vi "Tetra_TX-ATTEN_Payload.vi"(8 "error in":errorcluster, 10 "Input Constants":string[](array[string])=["18.75;1", "5;1", "COM4", "1", "1", "25", "0;0", "0;0", "1;20", "0", "0", "0", "", "10", "Z:\\State Files\\TEST2.csa", "", "3000", "4", "-10", "0.1", "", "", "C:\\RageATE\\Automated Tests\\Tetra WAM\\DVT\\Cal Files\\OUTPUT_CAL_080321-1118.csv"], 11 "Parameters":string[](array[string])=["skip", "18.75", "1", "5", "-1", "0", "5", "32.900000"]) -> (0 "error out":errorcluster, 2 "Payload Results":string[](array[string])=["-1.000", "-1.000", "32900.031", "-94.423", "-86.423", "-1.000", "16.450", "-1.000", "-1.000", "-1.000", "-1.000", "-1.000", "3.000", "-1.000", "-1.000", "15.000", "8.000", "8.000", "8.000", "-1.000", "-1.000", "-1.000", "-1.000", "-1.000", "-1.000", "-1.000", "-1.000", "-1.000", "-1.000", "-1.000", "-1.000", "-1.000", "-1.000", "-1.000", "-1.000", "-1.000", "-1.000", "-1.000", "-1.000", "-1.000", "-1.000", "-1.000", "-1.000", "-1.000", "0.504", "130.000", "-8.000", "32900.000", "-1.000", "-1.000", "P0027", "", "-1"])   [LabVIEW 2018]
uses:
  C:/RageATE-Tetra/Instruments/Ess Temp Plate/LabView Driver/Public/Watbus.dll
  Instruments/Ess Temp Plate/LabView Driver/Public/Watbus.dll
  8a334051-eedf-4406-ba3b-4766be56bf9e.vi
  458b4a15-084f-46bd-ad65-8d84519d0715.vi
  e7e3a4d5-9ed6-4285-8f90-f7af1205463a.vi
  778a857b-ea1c-4c41-85f0-8bde546241f8.vi
  765396e5-d7fa-4d1d-a6be-20604e030d46.vi
  35825170-2933-49a7-a6a3-6a45a8b9c174.vi
  498168d9-979f-4171-bbb2-b986919cd012.vi
  fd570da2-80e1-4258-b5ac-03cfe2f2c2d7.vi
  51f53847-2d88-46b1-9baf-ea88b261c08d.vi
  Initialize References/Station References Global.vi
  Initialize References/Sequence Globals.vi
  Tetra_Globals.vi
  Infrastructure/Test Parameter Globals_1.0.0.vi
  <vilib>/Utility/file.llb/Write Delimited Spreadsheet (DBL).vi
  <vilib>/Utility/file.llb/Read Delimited Spreadsheet (DBL).vi
  Instruments/Agilent N5232A PNA-L/Labview Driver/Keysight PNA Series/Keysight PNA Series.lvlib
  Instruments/PNA/lib functions/Agilent ENA Series.lvlib
panel:
  out "support_path":path
  out "RevC(t)":bool
  out "use-psa(t)":bool
  out "use-adar(t)":bool
  out "imon_pass?(t)":bool
  out "att_inl":dbl
  out "att_ref":dbl
  out "FiltRead":bool
  out "fault?(t)":bool
  in  "ess_error":errorcluster
  out "Freq Display":dbl=32.9 caption="Freq :  20"
  in  "Tab Control":T1(tab)
  out "MEAS_DCMON":bool
  out "CHIP_TEMP(t)":bool
  out "COMPORT":string="COM4"
  out "MODE":bool=TRUE
  out "Dist":dbl
  out "FILT_FCUT":dbl=25.0
  out "PLATE_TEMP(t)":bool
  out "MEAS_PS":bool
  out "MEAS_H2":bool=TRUE
  out "MEAS_Hx":bool=TRUE
  out "Hx_FREQ":dbl
  out "Hx_MULT":dbl
  out "H2_FREQ":dbl=40.0
  out "GANTRY(t)":bool=TRUE
  out "GET_DETECT":bool
  out "cmd;":string
  out "SOAK(m)":dbl
  out "Apply_FSL(t)":bool=TRUE
  out "MEAS_S11":bool
  out "S11_PORT":dbl
  out "comport":refnum<visa-resource-name>="COM4"
  out "AVG":i32=4
  out "ILabVIEW":refnum<k24>
  out "TEMP":dbl=25.0
  out "TX_PORT":i32=1
  out "V_SUPPLY":dbl=18.75
  out "EXT_ATT":dbl=5.0
  out "ADAR ATT":dbl
  out "TX_FILTER":i32=3
  out "REF_POW":dbl=5.0
  out "RF_FREQ":dbl=32.9
  out "TEMP(t)":bool
  out "V_SUPPLY(t)":bool
  out "TX_PORT(t)":bool
  out "REF_PWR(t)":bool
  out "TX_FILT(t)":bool
  out "ADAR_ATT(t)":bool
  out "EXT_ATT(t)":bool
  out "RF_FREQ(t)":bool=TRUE
  out "f_ref":dbl=16.45
  out "hx(t)":bool
  out "h2(t)":bool
  out "ps_meas(i)(w)":dbl[](array[numeric])=[-1.0, -1.0]
  out "rdv":dbl[](array[numeric])=[-1.0, -1.0, -1.0, -1.0, -1.0, -1.0, -1.0, -1.0, -1.0, -1.0]
  out "rdiv(i)":dbl[](array[numeric])=[-1.0, -1.0, -1.0, -1.0, -1.0, -1.0]
  out "rdiv(v)":dbl[](array[numeric])=[-1.0, -1.0, -1.0, -1.0, -1.0, -1.0]
  out "exa_mkr":dbl[](array[numeric])=[32900.0309, -94.423]
  out "h2_mkr":dbl[](array[numeric])=[-1.0, -1.0]
  out "Ampl_corr":dbl=-86.423
  out "s11":dbl=-1.0
  out "fsl_ampl_corr":dbl
  out "out_cal_ampl":dbl=-8.0
  out "out_cal freq":dbl=32900.0
  out "h2_dbc":dbl=-1.0
  out "hx_dbc":dbl
  out "hx_mkr":dbl[](array[numeric])
  out "fsl_corr_dB":dbl
  out "fsl(dB)":dbl
  out "att_dnl":dbl
  out "h2_lim":dbl
  out "out_cal":dbl[][](array[numeric])=[[0.0, 0.0], [20000.0, -6.076], [20100.0, -6.075], [20200.0, -6.219], [20300.0, -6.234], [20400.0, -6.315], [20500.0, -6.131], [20600.0, -6.004], [20700.0, -6.283], [20800.0, -6.485], [20900.0, -6.42], [21000.0, -6.941], [21100.0, -6.789], [21200.0, -6.508], [21300.0, -6.41], [21400.0, -6.872], [21500.0, -6.938], [21600.0, -7.017], [21700.0, -7.269], [21800.0, -6.683], [21900.0, -6.297], [22000.0, -6.38], [22100.0, -6.432], [22200.0, -6.851], [22300.0, -6.503], [22400.0, -6.961], [22500.0, -6.827], [22600.0, -6.62], [22700.0, -6.74], [22800.0, -6.547], [22900.0, -6.559], [23000.0, -6.434], [23100.0, -6.642], [23200.0, -6.654], [23300.0, -6.563], [23400.0, -6.6], [23500.0, -6.836], [23600.0, -6.685], [23700.0, -6.139], [23800.0, -6.472], [23900.0, -6.849], [24000.0, -6.765], [24100.0, -6.802], [24200.0, -6.636], [24300.0, -6.397], [24400.0, -6.33], [24500.0, -6.799], [24600.0, -6.985], [24700.0, -7.181], [24800.0, -7.304], [24900.0, -7.242], [25000.0, -7.104], [25100.0, -7.249], [25200.0, -7.246], [25300.0, -7.161], [25400.0, -7.073], [25500.0, -7.471], [25600.0, -7.347], [25700.0, -7.254], [25800.0, -7.048], [25900.0, -7.016], [26000.0, -7.055], [26100.0, -7.436], [26200.0, -7.416], [26300.0, -7.406], [26400.0, -7.616], [26500.0, -7.56], [26600.0, -7.304], [26700.0, -7.165], [26800.0, -7.047], [26900.0, -7.196], [27000.0, -8.144], [27100.0, -7.775], [27200.0, -7.683], [27300.0, -8.261], [27400.0, -7.702], [27500.0, -7.067], [27600.0, -7.418], [27700.0, -7.363], [27800.0, -7.557], [27900.0, -8.241], [28000.0, -7.789], [28100.0, -7.932], [28200.0, -7.422], [28300.0, -7.539], [28400.0, -7.363], [28500.0, -7.293], [28600.0, -7.623], [28700.0, -7.8], [28800.0, -7.603], [28900.0, -7.302], [29000.0, -7.428], [29100.0, -7.212], [29200.0, -7.395], [29300.0, -7.337], [29400.0, -7.17], [29500.0, -7.328], [29600.0, -7.393], [29700.0, -7.363], [29800.0, -7.396], [29900.0, -7.295], [30000.0, -7.448], [30100.0, -7.434], [30200.0, -7.524], [30300.0, -7.411], [30400.0, -7.422], [30500.0, -7.643], [30600.0, -7.707], [30700.0, -7.612], [30800.0, -7.742], [30900.0, -7.916], [31000.0, -7.904], [31100.0, -8.064], [31200.0, -8.185], [31300.0, -8.079], [31400.0, -8.102], [31500.0, -8.357], [31600.0, -7.974], [31700.0, -8.361], [31800.0, -8.902], [31900.0, -8.745], [32000.0, -8.522], [32100.0, -8.392], [32200.0, -8.221], [32300.0, -7.885], [32400.0, -8.215], [32500.0, -8.486], [32600.0, -8.735], [32700.0, -8.287], [32800.0, -8.037], [32900.0, -8.0], [33000.0, -7.651], [33100.0, -7.755], [33200.0, -8.158], [33300.0, -8.086], [33400.0, -8.531], [33500.0, -8.093], [33600.0, -7.791], [33700.0, -7.841], [33800.0, -8.085], [33900.0, -7.787], [34000.0, -7.696], [34100.0, -8.068], [34200.0, -8.028], [34300.0, -7.958], [34400.0, -7.778], [34500.0, -8.182], [34600.0, -7.565], [34700.0, -7.759], [34800.0, -7.899], [34900.0, -7.536], [35000.0, -7.873], [35100.0, -8.126], [35200.0, -8.061], [35300.0, -7.731], [35400.0, -7.575], [35500.0, -7.802], [35600.0, -7.335], [35700.0, -7.39], [35800.0, -7.975], [35900.0, -7.981], [36000.0, -7.422], [36100.0, -7.632], [36200.0, -8.267], [36300.0, -7.907], [36400.0, -7.609], [36500.0, -7.858], [36600.0, -8.426], [36700.0, -8.44], [36800.0, -8.438], [36900.0, -8.536], [37000.0, -8.361], [37100.0, -8.731], [37200.0, -8.549], [37300.0, -8.609], [37400.0, -8.746], [37500.0, -9.42], [37600.0, -9.062], [37700.0, -8.792], [37800.0, -8.948], [37900.0, -8.893], [38000.0, -9.551], [38100.0, -9.086], [38200.0, -8.754], [38300.0, -8.61], [38400.0, -8.629], [38500.0, -8.895], [38600.0, -8.79], [38700.0, -8.437], [38800.0, -8.982], [38900.0, -8.564], [39000.0, -8.456], [39100.0, -8.944], [39200.0, -9.606], [39300.0, -9.246], [39400.0, -9.208], [39500.0, -9.78], [39600.0, -9.779], [39700.0, -9.292], [39800.0, -9.924], [39900.0, -9.871], [40000.0, -9.839]]
  out "h2_cal_ampl":dbl=-1.0
  out "h2_cal freq":dbl=-1.0
  out "h2_corr":dbl=-1.0
  out "h2_fsl_corr":dbl
  out "hx_cal_ampl":dbl=-1.0
  out "hx_cal freq":dbl=-1.0
  out "hx_fsl_corr":dbl
  out "hx_corr":dbl
  out "horn_Cal Freq Out":dbl
  out "horn_Ampl Out":dbl
  out "horn_cal":dbl[][](array[numeric])
  out "bpf":i32=1
  out "temp 0x":string="-1"
  out "detect":dbl=-1.0
  out "filt(num)":i32=3
  out "txatten-sel":i32=-1
  out "ext-atten(val)":dbl=-1.0
  out "adar-att(val)":dbl=-1.0
  out "iteration time(s)":dbl=91659.4314544 format="%_19f"
  out "relative seconds":dbl=91658.92763549999 format="%_19f"
  out "x-y":dbl=0.1592017999937525
  out "atten(code)ary (ro)":i32[](array[numeric])=[15, 8, 8, 8]
  out "plate_temp":sgl[](array[numeric])=[-1.0, -1.0] format="%.3g"
  out "temp_data":dbl[](array[numeric])
  out "dcw_lsl":dbl
  out "dcw_hsl":dbl
  out "pout_lsl":dbl
  out "pout_hsl":dbl
  out "s11_lsl":dbl
  out "s11_hsl":dbl
  out "FH_NOT(T)":bool
  out "no_fault":bool
  out "STOP(T)":bool
  # "Constants Locals Used in Payload"
  # "Index\tKey\tInput Constants\tUnits\n0\t1\tPS1-1 V;I\tVolt : Amp\n1\t1\tPS1-2 V:I\tVolt : Amp\n2\t1\tCOM PORT\tSTR\n3\t1\tMODE\tBool\n4\t1\tTXPORT;Antenna Dist\tant/inch\n5\t1\tTX Filt Cutoff\tGHz\n6\t1\tMeas Plate Temp; Meas Chip Temp\tBool;Bool\n7\t1\tMeas DC PS;Meas DCMON (Chip)\tBool;Bool\n8\t1\tMeas H2 \tBool;Freq(GHz)\n9\t1\tMeas H*x\tFreq(GHz);multiplier\n10\t1\tMeas S11;TXPORT\tBool;num\n11\t1\tRead Detector (1-4) \tBool\n12\t1\tcmd;…\tcmd;cmd\n13\t1\tTemp Soak Time\tmin\n14\t1\tPNA State File (local)\tPath\n15\t1\tENA State File\tPath\n16\t1\tENA RBW\tHz\n17\t1\tENA #of AVGs\tnum\n18\t1\tENA Ref Lvl\tdB\n19\t1\tENA Span\tMHz\n20\t1\tRFIN_CAL\tpath\n21\t1\tHORN_CAL\tpath\n22\t1\tOUTPUT_CAL\tpath\n23\t1\tFSL_APPLY\tbool\n24\t1\tDCW_LIMITS\tlsl;hsl\n25\t1\tPOUT_LIMITS\tlsl;hsl\n26\t1\tS11_LIMITS\tlsl;hsl"
  # "Input Parameters Locals"
  # "Update(t)"
  # "TEMP\nPS1-1_V\nRF_FREQ_OUT\nTX_PORT\nTX_FILT\nADAR_ATT\nPSA_ATT\nREF_POWER"
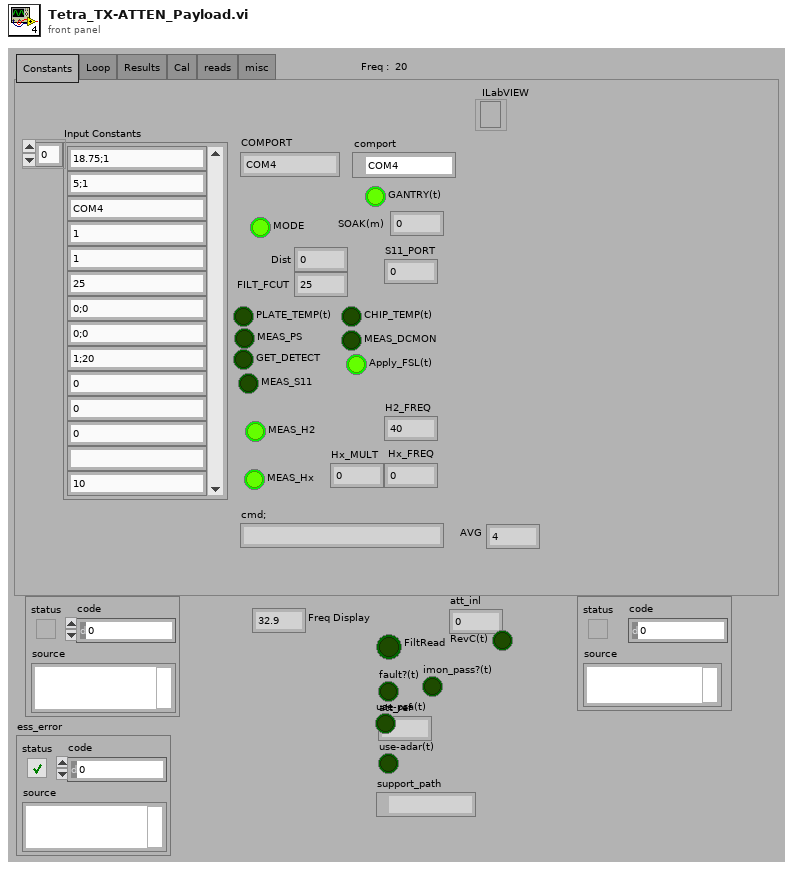
[diagram p1: front panel]
types:
  T1 = enum32{"Constants", "Loop", "Results", "Cal", "reads", "misc"}
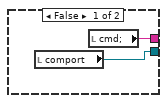
[diagram p2: hidden frame]
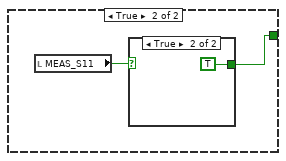
[diagram p3: hidden frame]
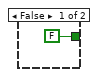
[diagram p4: hidden frame]
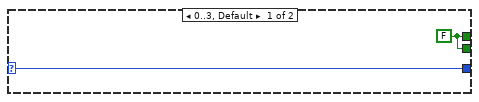
[diagram p5: hidden frame]
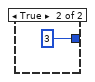
[diagram p6: hidden frame]
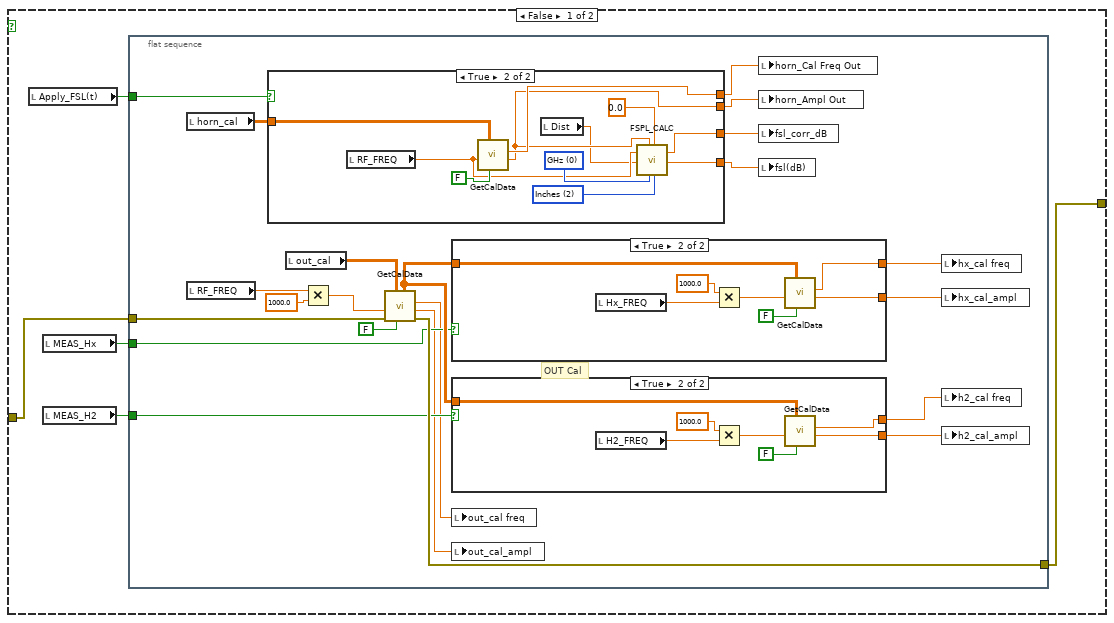
[diagram p7: hidden frame]
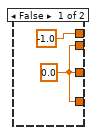
[diagram p8: hidden frame]
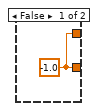
[diagram p9: hidden frame]
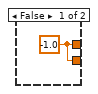
[diagram p10: hidden frame]
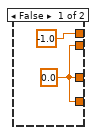
[diagram p11: hidden frame]
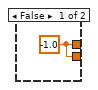
[diagram p12: hidden frame]
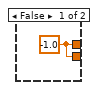
[diagram p13: hidden frame]
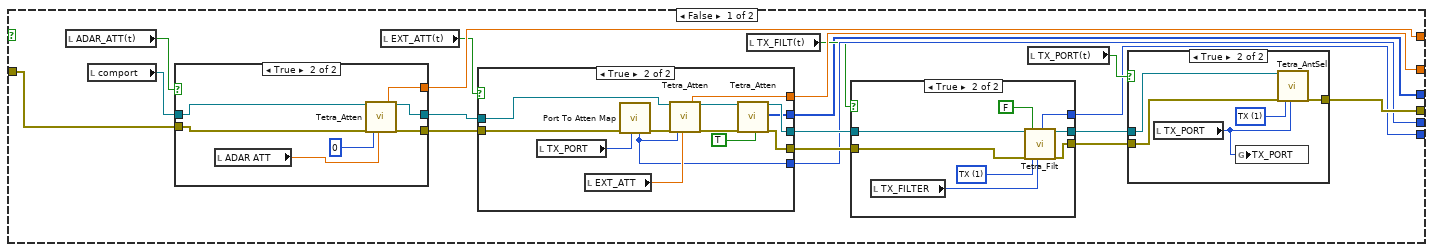
[diagram p17: hidden frame]
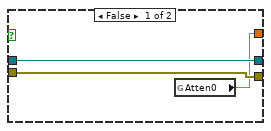
[diagram p18: hidden frame]
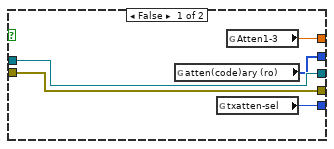
[diagram p19: hidden frame]
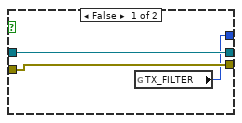
[diagram p20: hidden frame]
diagram:
  n1 = flat-sequence {
    tunnel: ["error in"] -> w11
    tunnel: [w24] -> w1
    tunnel: [w37] -> w13
    tunnel: [w36] -> w12
    tunnel: w11 -> [w35]
    tunnel: w1 -> [w33]
    tunnel: [w956] -> w14
    tunnel: [w941] -> w15
    tunnel: [w959] -> w16
    tunnel: [w960] -> w18
    tunnel: w13 -> [w960]
    tunnel: w12 -> [w959]
    tunnel: [w958] -> w10
    tunnel: [w957] -> w9
    tunnel: [w945] -> w6
    tunnel: [w955] -> w8
    tunnel: [w952] -> w7
    frame #0 {
      n2 = flat-sequence {
        frame #0 {
          w28 = TRUE ("Test Running (T)")
          n3 = global read "Station References Global.vi" "Gantry"() -> (w29:refnum<visa-resource-name>)
          n4 = call "WAM_ESS.vi"("VISA resource name"=w29, "error in (no error)"="ess_error", "Open Serial"=w28, "Test Running (T)"=w28, "Close Serial"=w28) -> ("FH_NOT(T)"=→"FH_NOT(T)":bool, "error out"=w26:errorcluster)  [unwired: 7 in, 2 out]
          n5 = local write "ess_error"(w26) -> ()
        }
      }
      n6 = global read "Sequence Globals.vi" "AppSupportPath"() -> (w20:path)
      n7 = global read "Sequence Globals.vi" "DevSupportPath"() -> (w21:path)
      n8 = global read "Tetra_Globals.vi" "RevC(t)"() -> (→"RevC(t)":bool)
      n9 = global read "Sequence Globals.vi" "IsRuntime?"() -> (w22:bool)
      n10 = Select(t=w20, s=w22, f=w21) -> (s? t:f=→"support_path":path)
      n11 = global read "Sequence Globals.vi" "Stop Testing"() -> (w24:bool)
    }
    frame #1 {
      n12 = Select(t=0, s=w33, f=2) -> (s? t:f=w34:i32)
      n13 = for {
        N: w34 -> [_]
        tunnel: [w46] -> w37
        tunnel: [w45] -> w36
        tunnel: w35 -> [w44]
        i -> [w41]
        stop <- w39 stop-if-true
        n14 = flat-sequence {
          tunnel: [w79] -> w78
          tunnel: ["Parameters"] -> w77
          tunnel: ["Input Constants"] -> w76
          tunnel: w44 -> [w79]
          tunnel: w78 -> [w85]
          tunnel: [w84] -> w75
          tunnel: w77 -> [w97]
          tunnel: w76 -> [w96]
          tunnel: [w95] -> w74
          tunnel: [w94] -> w73
          tunnel: [w93] -> w72
          tunnel: [w83] -> w71
          tunnel: [w92] -> w70
          tunnel: [w90] -> w69
          tunnel: [w91] -> w68
          tunnel: [w89] -> w67
          tunnel: [w88] -> w66
          tunnel: [w87] -> w65
          tunnel: w75 -> [w234]
          tunnel: [w234] -> w64
          tunnel: w74 -> [w233]
          tunnel: w73 -> [w230]
          tunnel: w72 -> [w218]
          tunnel: w71 -> [w213]
          tunnel: w70 -> [w227]
          tunnel: w69 -> [w226]
          tunnel: w68 -> [w224]
          tunnel: w67 -> [w221]
          tunnel: w66 -> [w219]
          tunnel: w65 -> [w211]
          tunnel: w64 -> [w277]
          tunnel: [w276] -> w63
          tunnel: [w391] -> w62
          tunnel: w63 -> [w390]
          tunnel: w62 -> [w407]
          tunnel: [w407] -> w61
          tunnel: w61 -> [w409]
          tunnel: [w409] -> w43
          tunnel: [w424] -> w60
          tunnel: w43 -> [w424]
          tunnel: w60 -> [w425]
          tunnel: [w426] -> w59
          tunnel: w59 -> [w438]
          tunnel: [w438] -> w58
          tunnel: [w437] -> w57
          tunnel: [w441] -> w56
          tunnel: w58 -> [w440]
          tunnel: w57 -> [w439]
          tunnel: [w439] -> w55
          tunnel: w56 -> [w572]
          tunnel: [w572] -> w54
          tunnel: w55 -> [w570]
          tunnel: [w574] -> w53
          tunnel: w54 -> [w573]
          tunnel: w53 -> [w596]
          tunnel: [w596] -> w52
          tunnel: w52 -> [w602]
          tunnel: [w597] -> w51
          tunnel: [w746] -> w50
          tunnel: w51 -> [w748]
          tunnel: w50 -> [w843]
          tunnel: [w843] -> w49
          tunnel: [w845] -> w48
          tunnel: w49 -> [w844]
          tunnel: w48 -> [w872]
          tunnel: [w872] -> w47
          tunnel: [w871] -> w42
          tunnel: [w908] -> w46
          tunnel: w47 -> [w898]
          tunnel: [w898] -> w45
          tunnel: [w896] -> w38
          frame #0 {
            n15 = call <vilib>:"High Resolution Relative Seconds.vi"() -> ("relative seconds"=→"relative seconds":dbl)
          }
          frame #1 {
            # "TEMP\nPS1-1_V\nRF_FREQ_OUT\nTX_PORT\nTX_FILT\nADAR_ATT\nPSA_ATT\nREF_POWER"
            n16 = flat-sequence {
              tunnel: w96 -> [w197]
              tunnel: [w165] -> w87
              frame #0 {
                # "Get the Test Constants"
                n17 = Index Array(array=w197, index #1=2 ("index"), index #3=4 ("index"), index #8=10 ("index"), index #10=17 ("index"), index #11=20 ("index"), index #12=9 ("index"), index #13=13 ("index"), index #14=23 ("index")) -> (element #1=→"COMPORT":string, element #2=w172:string, element #3=w147:string, element #4=w187:string, element #5=w191:string, element #6=w190:string, element #7=w180:string, element #8=w169:string, element #9=w181:string, element #10=w182:string, element #12=w163:string, element #13=w152:string, element #14=w148:string, element #15=w139:string, element #16=w142:string, element #17=w134:string, element #18=w128:string)  [unwired: 10 in, 1 out]
                n18 = call "StringToNumberControlWithBool.vi"("String In"=w172) -> ("NOT = 0"=→"MODE":bool)  [unwired: 7 in, 1 out]
                n19 = call "StringToNumberControlWithBool.vi"("String In"=w152) -> ("Number Out"=→"SOAK(m)":dbl)  [unwired: 7 in, 1 out]
                n20 = call <vilib>:"Trim Whitespace.vi"("string"=w163) -> ("trimmed string"=w159:string)  [unwired: 1 in]
                n21 = call "StringToNumberControlWithBool.vi"("String In"=w182) -> ("Number Out"=→"AVG":dbl)  [unwired: 7 in, 1 out]
                n22 = Match Pattern(string=w147, regular expression=";") -> (before substring=w146:string, after substring=w144:string)  [unwired: 1 in, 2 out]
                n23 = call "StringToNumberControlWithBool.vi"("String In"=w187) -> ("Number Out"=→"FILT_FCUT":dbl)  [unwired: 7 in, 1 out]
                n24 = Match Pattern(string=w191, regular expression=";") -> (before substring=w195:string, after substring=w194:string)  [unwired: 1 in, 2 out]
                n25 = Match Pattern(string=w190, regular expression=";") -> (before substring=w203:string, after substring=w202:string)  [unwired: 1 in, 2 out]
                n26 = Match Pattern(string=w180, regular expression=";") -> (before substring=w178:string, after substring=w176:string)  [unwired: 1 in, 2 out]
                n27 = Match Pattern(string=w169, regular expression=";") -> (before substring=w168:string, after substring=w166:string)  [unwired: 1 in, 2 out]
                n28 = Match Pattern(string=w159, regular expression=";") -> (before substring=w162:string, after substring=w161:string)  [unwired: 1 in, 2 out]
                n29 = call "StringToNumberControlWithBool.vi"("String In"=w146) -> ("NOT = 0"=→"GANTRY(t)":bool)  [unwired: 7 in, 1 out]
                n30 = call "StringToNumberControlWithBool.vi"("String In"=w144) -> ("Number Out"=→"Dist":dbl)  [unwired: 7 in, 1 out]
                n31 = call "StringToNumberControlWithBool.vi"("String In"=w195) -> ("NOT = 0"=→"PLATE_TEMP(t)":bool)  [unwired: 7 in, 1 out]
                n32 = call "StringToNumberControlWithBool.vi"("String In"=w203) -> ("NOT = 0"=→"MEAS_PS":bool)  [unwired: 7 in, 1 out]
                n33 = call "StringToNumberControlWithBool.vi"("String In"=w194) -> ("NOT = 0"=→"CHIP_TEMP(t)":bool)  [unwired: 7 in, 1 out]
                n34 = call "StringToNumberControlWithBool.vi"("String In"=w202) -> ("NOT = 0"=→"MEAS_DCMON":bool)  [unwired: 7 in, 1 out]
                n35 = call "StringToNumberControlWithBool.vi"("String In"=w178) -> ("NOT = 0"=→"MEAS_H2":bool)  [unwired: 7 in, 1 out]
                n36 = call "StringToNumberControlWithBool.vi"("String In"=w176) -> ("Number Out"=→"H2_FREQ":dbl)  [unwired: 7 in, 1 out]
                n37 = call "StringToNumberControlWithBool.vi"("String In"=w168) -> ("NOT = 0"=→"MEAS_S11":bool)  [unwired: 7 in, 1 out]
                n38 = call "StringToNumberControlWithBool.vi"("String In"=w148) -> ("NOT = 0"=→"Apply_FSL(t)":bool)  [unwired: 7 in, 1 out]
                n39 = call "StringToNumberControlWithBool.vi"("String In"=w181) -> ("NOT = 0"=→"GET_DETECT":bool)  [unwired: 7 in, 1 out]
                n40 = call "StringToNumberControlWithBool.vi"("String In"=w166) -> ("Number Out"=→"S11_PORT":dbl)  [unwired: 7 in, 1 out]
                n41 = call "StringToNumberControlWithBool.vi"("String In"=w162) -> ("Number Out"=→"Hx_FREQ":dbl, "NOT = 0"=w158:bool)  [unwired: 7 in]
                n42 = call "StringToNumberControlWithBool.vi"("String In"=w161) -> ("Number Out"=→"Hx_MULT":dbl, "NOT = 0"=w157:bool)  [unwired: 7 in]
                n43 = call "StringToNumberControlWithBool(x2).vi"("Seperator"=";" ("regular expression"), "string"=w139) -> ("Num(2)"=→"dcw_hsl":dbl, "Num"=→"dcw_lsl":dbl, "Seperator Out"=w135:string)  [unwired: 3 in, 4 out]
                n44 = call "StringToNumberControlWithBool(x2).vi"("Seperator"=w135, "string"=w142) -> ("Num(2)"=→"pout_hsl":dbl, "Num"=→"pout_lsl":dbl, "Seperator Out"=w133:string)  [unwired: 3 in, 4 out]
                n45 = call "StringToNumberControlWithBool(x2).vi"("Seperator"=w133, "string"=w134) -> ("Num(2)"=→"s11_hsl":dbl, "Num"=→"s11_lsl":dbl, "Seperator Out"=w130:string)  [unwired: 3 in, 4 out]
                n46 = call "StringToNumberControlWithBool(x2).vi"("Seperator"=w130, "string"=w128) -> ("Num"=→"h2_lim":dbl)  [unwired: 3 in, 6 out]
                n47 = And(x=w158, y=w157) -> (x .and. y?=→"MEAS_Hx":bool)
                n48 = Empty String/Path?(string/path=w166) -> (empty?=w165:bool)
              }
            }
            n49 = control-ref of="Freq Display"() -> (w86:refnum<vi>)
            n50 = flat-sequence {
              tunnel: w97 -> [w125]
              tunnel: [w98] -> w95
              tunnel: [w103] -> w94
              tunnel: [w124] -> w93
              tunnel: [w123] -> w83
              tunnel: [w122] -> w92
              tunnel: [w121] -> w91
              tunnel: [w120] -> w90
              tunnel: [w118] -> w89
              tunnel: [w113] -> w88
              tunnel: w86 -> [w112]
              tunnel: w85 -> [w109]
              tunnel: [w108] -> w84
              frame #0 {
                # "Get the Test Parameters"
                n51 = Index Array(array=w125) -> (element #1=w120:string, element #2=w126:string, element #3=w106:string, element #4=w104:string, element #5=w117:string, element #6=w116:string, element #7=w107:string, element #8=w105:string)  [unwired: 8 in]
                n52 = Concatenate Strings("Freq :  " ("string"), w106) -> (w111:string)
                n53 = call "TempControlWithBool.vi"("INPUT"=w120) -> ("out"=→"TEMP":dbl, "Valid(t)"=w118:bool)  [unwired: 6 in, 1 out]
                n54 = Fract/Exp String To Number(string=w126) -> (number=w122:dbl)  [unwired: 3 in, 1 out]
                "V_SUPPLY" <- w122
                n55 = Decimal String To Number(string=w104) -> (number=w123:i32)  [unwired: 2 in, 1 out]
                "TX_PORT" <- w123
                n56 = Decimal String To Number(string=w117) -> (number=w124:i32)  [unwired: 2 in, 1 out]
                "TX_FILTER" <- w124
                n57 = Fract/Exp String To Number(string=w116) -> (number=w103:dbl)  [unwired: 3 in, 1 out]
                "ADAR ATT" <- w103
                n58 = Fract/Exp String To Number(string=w107) -> (number=w98:dbl)  [unwired: 3 in, 1 out]
                "EXT_ATT" <- w98
                n59 = Fract/Exp String To Number(string=w105) -> (number=w121:dbl)  [unwired: 3 in, 1 out]
                "REF_POW" <- w121
                n60 = Fract/Exp String To Number(string=w106) -> (number=w113:dbl)  [unwired: 3 in, 1 out]
                "RF_FREQ" <- w113
                "Freq Display" <- w113
                n61 = property class="DigNum (strict)"(reference=w112, error in=w109, "Caption.Text"=w111) -> (error out=w108:errorcluster)  [unwired: 1 out]
                n62 = Divide(x=w113, y=2.0) -> (x/y=→"f_ref":dbl)
                n63 = Not Equal?(x=w98, y=-1.0) -> (x != y?=→"use-psa(t)":bool)
                n64 = Not Equal?(x=w103, y=-1.0) -> (x != y?=→"use-adar(t)":bool)
              }
            }
          }
          frame #2 {
            # "Check if value changed\nif value changed (t) use to skip the routine"
            n65 = call "Is Value Changed.vim"("value"=w226) -> ("changed or first call?"=w223:bool)
            n66 = call "Is Value Changed.vim"("value"=w227) -> ("changed or first call?"=→"V_SUPPLY(t)":bool)
            n67 = call "Is Value Changed.vim"("value"=w219) -> ("changed or first call?"=→"RF_FREQ(t)":bool)
            n68 = call "Is Value Changed.vim"("value"=w213) -> ("changed or first call?"=→"TX_PORT(t)":bool)
            n69 = call "Is Value Changed.vim"("value"=w230) -> ("changed or first call?"=→"ADAR_ATT(t)":bool)
            n70 = call "Is Value Changed.vim"("value"=w233) -> ("changed or first call?"=→"EXT_ATT(t)":bool)
            n71 = call "Is Value Changed.vim"("value"=w224) -> ("changed or first call?"=→"REF_PWR(t)":bool)
            n72 = flat-sequence {
              frame #0 {
                # "Setup the H*X measurement"
                n73 = local read "MEAS_Hx"() -> (w245:bool)
                n74 = local read "Hx_MULT"() -> (w242:dbl)
                n75 = local read "Hx_FREQ"() -> (w244:dbl)
                n76 = local read "RF_FREQ"() -> (w248:dbl)
                n77 = Equal?(x=w244, y=w248) -> (x = y?=w247:bool)
                n78 = Multiply(x=w244, y=w242) -> (x*y=w243:dbl)
                n79 = local write "Hx_FREQ"(w243) -> ()
                n80 = And(x=w247, y=w245) -> (x .and. y?=→"hx(t)":bool)
              }
            }
            n81 = flat-sequence {
              frame #0 {
                # "Setup the H2 measurement"
                n82 = local read "H2_FREQ"() -> (w260:dbl)
                n83 = Multiply(x=w260, y=2.0) -> (x*y=w258:dbl)
                n84 = local write "H2_FREQ"(w258) -> ()
                n85 = local read "RF_FREQ"() -> (w264:dbl)
                n86 = local read "MEAS_H2"() -> (w261:bool)
                n87 = Equal?(x=w260, y=w264) -> (x = y?=w263:bool)
                n88 = And(x=w263, y=w261) -> (x .and. y?=→"h2(t)":bool)
              }
            }
            n89 = case shown="-1" w218 {
              selector: w218 -> [w266 _]
              tunnel: [w266 w269] -> w217
              tunnel: [w265 w268] -> w214
              tunnel: [w265 TRUE ("TX_FILT(t) 2")] -> w205
              frame 0..3, Default {
                w265 = FALSE ("changed or first call?")
              }
              frame -1 {
                n90 = local read "FILT_FCUT"() -> (w271:dbl)
                n91 = local read "RF_FREQ"() -> (w272:dbl)
                n92 = Greater Or Equal?(x=w272, y=w271) -> (x >= y?=w270:bool)
                n93 = case shown="False" w270 {
                  tunnel: [2 3] -> w269
                  frame False {
                  }
                  frame True {
                  }
                }
                n94 = call "Is Value Changed.vim"("value"=w269) -> ("changed or first call?"=w268:bool)
              }
            }
            "FiltRead" <- w205
            n95 = local read "MEAS_S11"() -> (w209:bool)
            n96 = First Call?() -> (First Call?: T/F=w207:bool)
            n97 = case shown="True" w207 {
              tunnel: [w236 w241] -> w206
              tunnel: [w235 w238] -> w208
              frame False {
                n98 = local read "comport"() -> (w235:refnum<visa-resource-name>)
                n99 = local read "cmd;"() -> (w236:string)
              }
              frame True {
                n100 = local read "COMPORT"() -> (w237:string)
                n101 = global read "Tetra_Globals.vi" "comport"() -> (w239:refnum<visa-resource-name>)
                n102 = Empty String/Path?(string/path=w237) -> (empty?=w240:bool)
                n103 = global read "Tetra_Globals.vi" "cmd;"() -> (w241:string)
                n104 = Select(t=w239, s=w240, f=w237) -> (s? t:f=w238:refnum<visa-resource-name>)
              }
            }
            "cmd;" <- w206
            "comport" <- w208
            n105 = And(x=w223, y=w221) -> (x .and. y?=→"TEMP(t)":bool)
            n106 = And(x=w211, y=w209) -> (x .and. y?=w210:bool)
            n107 = case shown="False" w210 {
              tunnel: w213 -> [w253 _]
              tunnel: [w249 w255] -> w212
              frame False {
                n108 = local read "S11_PORT"() -> (w252:dbl)
                n109 = local read "MEAS_S11"() -> (w250:bool)
                n110 = Equal?(x=w252, y=w253) -> (x = y?=w251:bool)
                n111 = And(x=w250, y=w251) -> (x .and. y?=w249:bool)
              }
              frame True {
                n112 = local read "MEAS_S11"() -> (w254:bool)
                n113 = case shown="True" w254 {
                  tunnel: [FALSE TRUE] -> w255
                  frame False {
                  }
                  frame True {
                  }
                }
              }
            }
            n114 = call "Is Value Changed.vim"("value"=w218) -> ("changed or first call?"=w215:bool)
            n115 = Or(x=w214, y=w215) -> (x .or. y?=→"TX_FILT(t)":bool)
            n116 = local write "TX_FILTER"(w217) -> ()
            n117 = local write "MEAS_S11"(w212) -> ()
          }
          frame #3 {
            # "Need to reorganize cal and off load to the instruments"
            # "Read the global cal-Write to locals\n-Use locals after 1sT iteration"
            n118 = First Call?() -> (First Call?: T/F=w275:bool)
            n119 = case shown="True" w275 {
              tunnel: w277 -> [w282 w338]
              tunnel: [w281 w337] -> w276
              frame False {
                n120 = local read "Apply_FSL(t)"() -> (w278:bool)
                n121 = local read "MEAS_Hx"() -> (w279:bool)
                n122 = local read "MEAS_H2"() -> (w280:bool)
                n123 = flat-sequence {
                  tunnel: [w301] -> w281
                  tunnel: w282 -> [w302]
                  tunnel: w280 -> [w298]
                  tunnel: w279 -> [w296]
                  tunnel: w278 -> [w295]
                  frame #0 {
                    # "OUT Cal"
                    n124 = local read "horn_cal"() -> (w287:dbl[][])
                    n125 = local read "RF_FREQ"() -> (w304:dbl)
                    n126 = case shown="True" w295 {
                      tunnel: [-1.0 ("Cal Freq Out") w316] -> w286
                      tunnel: [w305 w315] -> w285
                      tunnel: w287 -> [_ w314]
                      tunnel: [w305 w310] -> w284
                      tunnel: [w305 w308] -> w283
                      frame False {
                        w305 = 0.0 ("Ampl Out")
                      }
                      frame True {
                        w311 = u16 2 items=["Meter", "Feet", "Inches"] ("d(units)")
                        w313 = u16 0 items=["GHz", "MHz"] ("f(units)")
                        n127 = local read "RF_FREQ"() -> (w309:dbl)
                        n128 = call "GetCalData.vi"("Open new file T"=FALSE, "Ary In"=w314, "RF Freq (MHz)"=w309) -> ("Ampl Out"=w315:dbl, "Cal Freq Out"=w316:dbl)  [unwired: 3 in, 4 out]
                        n129 = local read "Dist"() -> (w307:dbl)
                        n130 = call "FSPL_CALC.vi"("f"=w309, "d"=w307, "Ant1 Gain (dB)"=w315, "f(units)"=w313, "Ant2 Gain dB"=0.0 ("Ant1 Gain (dB)"), "d(units)"=w311) -> ("Corr(dB)"=w310:dbl, "fsl(dB)"=w308:dbl)  [unwired: 11 in, 1 out]
                      }
                    }
                    n131 = local read "out_cal"() -> (w294:dbl[][])
                    n132 = Multiply(x=w304, y=1000.0) -> (x*y=w303:dbl)
                    n133 = call "GetCalData.vi"("Open new file T"=FALSE, "Ary In"=w294, "error in (no error)"=w302, "RF Freq (MHz)"=w303) -> ("error out"=w301:errorcluster, "Ampl Out"=w292:dbl, "Cal Freq Out"=w293:dbl, "array out"=w297:dbl[][])  [unwired: 2 in, 2 out]
                    n134 = case shown="True" w296 {
                      tunnel: [w318 w324] -> w289
                      tunnel: [w318 w323] -> w288
                      tunnel: w297 -> [_ w321]
                      frame False {
                        w318 = -1.0 ("Ampl Out")
                      }
                      frame True {
                        n135 = local read "Hx_FREQ"() -> (w325:dbl)
                        n136 = Multiply(x=1000.0 ("y"), y=w325) -> (x*y=w322:dbl)
                        n137 = call "GetCalData.vi"("Open new file T"=FALSE, "Ary In"=w321, "RF Freq (MHz)"=w322) -> ("Ampl Out"=w323:dbl, "Cal Freq Out"=w324:dbl)  [unwired: 3 in, 4 out]
                      }
                    }
                    n138 = case shown="True" w298 {
                      tunnel: [w326 w332] -> w290
                      tunnel: [w326 w331] -> w291
                      tunnel: w297 -> [_ w329]
                      frame False {
                        w326 = -1.0 ("Ampl Out")
                      }
                      frame True {
                        n139 = local read "H2_FREQ"() -> (w333:dbl)
                        n140 = Multiply(x=1000.0 ("y"), y=w333) -> (x*y=w330:dbl)
                        n141 = call "GetCalData.vi"("Open new file T"=FALSE, "Ary In"=w329, "RF Freq (MHz)"=w330) -> ("Ampl Out"=w331:dbl, "Cal Freq Out"=w332:dbl)  [unwired: 3 in, 4 out]
                      }
                    }
                    n142 = local write "out_cal freq"(w293) -> ()
                    n143 = local write "out_cal_ampl"(w292) -> ()
                    n144 = local write "horn_Cal Freq Out"(w286) -> ()
                    n145 = local write "horn_Ampl Out"(w285) -> ()
                    n146 = local write "fsl_corr_dB"(w284) -> ()
                    n147 = local write "fsl(dB)"(w283) -> ()
                    n148 = local write "hx_cal freq"(w289) -> ()
                    n149 = local write "hx_cal_ampl"(w288) -> ()
                    n150 = local write "h2_cal freq"(w290) -> ()
                    n151 = local write "h2_cal_ampl"(w291) -> ()
                  }
                }
              }
              frame True {
                n152 = local read "Apply_FSL(t)"() -> (w334:bool)
                n153 = local read "MEAS_Hx"() -> (w335:bool)
                n154 = local read "MEAS_H2"() -> (w336:bool)
                n155 = flat-sequence {
                  tunnel: [w355] -> w337
                  tunnel: w338 -> [w356]
                  tunnel: w336 -> [w349]
                  tunnel: w335 -> [w345]
                  tunnel: w334 -> [w342]
                  frame #0 {
                    # "OUT Cal"
                    n156 = global read "Tetra_Globals.vi" "HORN_CAL"() -> (w343:dbl[][])
                    "horn_cal" <- w343
                    n157 = local read "RF_FREQ"() -> (w360:dbl)
                    n158 = case shown="True" w342 {
                      tunnel: [-1.0 ("Cal Freq Out") w372] -> w344
                      tunnel: [w361 w371] -> w341
                      tunnel: w343 -> [_ w370]
                      tunnel: [w361 w366] -> w340
                      tunnel: [w361 w364] -> w339
                      frame False {
                        w361 = 0.0 ("Ampl Out")
                      }
                      frame True {
                        w367 = u16 2 items=["Meter", "Feet", "Inches"] ("d(units)")
                        w369 = u16 0 items=["GHz", "MHz"] ("f(units)")
                        n159 = local read "RF_FREQ"() -> (w365:dbl)
                        n160 = call "GetCalData.vi"("Open new file T"=FALSE, "Ary In"=w370, "RF Freq (MHz)"=w365) -> ("Ampl Out"=w371:dbl, "Cal Freq Out"=w372:dbl)  [unwired: 3 in, 4 out]
                        n161 = local read "Dist"() -> (w363:dbl)
                        n162 = call "FSPL_CALC.vi"("f"=w365, "d"=w363, "Ant1 Gain (dB)"=w371, "f(units)"=w369, "Ant2 Gain dB"=0.0 ("Ant1 Gain (dB)"), "d(units)"=w367) -> ("Corr(dB)"=w366:dbl, "fsl(dB)"=w364:dbl)  [unwired: 11 in, 1 out]
                      }
                    }
                    "horn_Cal Freq Out" <- w344
                    "horn_Ampl Out" <- w341
                    "fsl_corr_dB" <- w340
                    "fsl(dB)" <- w339
                    n163 = global read "Tetra_Globals.vi" "OUT_CAL"() -> (w352:dbl[][])
                    "out_cal" <- w352
                    n164 = Multiply(x=w360, y=1000.0) -> (x*y=w359:dbl)
                    n165 = call "GetCalData.vi"("Open new file T"=FALSE, "Ary In"=w352, "error in (no error)"=w356, "RF Freq (MHz)"=w359) -> ("error out"=w355:errorcluster, "Ampl Out"=→"out_cal_ampl":dbl, "Cal Freq Out"=→"out_cal freq":dbl, "array out"=w346:dbl[][])  [unwired: 2 in, 2 out]
                    n166 = case shown="True" w345 {
                      tunnel: [w374 w380] -> w347
                      tunnel: [w374 w379] -> w348
                      tunnel: w346 -> [_ w377]
                      frame False {
                        w374 = -1.0 ("Ampl Out")
                      }
                      frame True {
                        n167 = local read "Hx_FREQ"() -> (w381:dbl)
                        n168 = Multiply(x=1000.0 ("y"), y=w381) -> (x*y=w378:dbl)
                        n169 = call "GetCalData.vi"("Open new file T"=FALSE, "Ary In"=w377, "RF Freq (MHz)"=w378) -> ("Ampl Out"=w379:dbl, "Cal Freq Out"=w380:dbl)  [unwired: 3 in, 4 out]
                      }
                    }
                    "hx_cal freq" <- w347
                    "hx_cal_ampl" <- w348
                    n170 = case shown="True" w349 {
                      tunnel: [w382 w388] -> w351
                      tunnel: [w382 w387] -> w350
                      tunnel: w346 -> [_ w385]
                      frame False {
                        w382 = -1.0 ("Ampl Out")
                      }
                      frame True {
                        n171 = local read "H2_FREQ"() -> (w389:dbl)
                        n172 = Multiply(x=1000.0 ("y"), y=w389) -> (x*y=w386:dbl)
                        n173 = call "GetCalData.vi"("Open new file T"=FALSE, "Ary In"=w385, "RF Freq (MHz)"=w386) -> ("Ampl Out"=w387:dbl, "Cal Freq Out"=w388:dbl)  [unwired: 3 in, 4 out]
                      }
                    }
                    "h2_cal freq" <- w351
                    "h2_cal_ampl" <- w350
                  }
                }
              }
            }
          }
          frame #4 {
            n174 = flat-sequence {
              tunnel: [w395] -> w391
              tunnel: w390 -> [w394]
              frame #0 {
                # "3-23-22\nneed to add bypass if ess is tripped so it wont set the temperature and soak"
                # "Set The Temperature"
                n175 = global read "Station References Global.vi" "Oven Present?"() -> (w392:bool)
                n176 = local read "TEMP(t)"() -> (w396:bool)
                n177 = And(x=w396, y=w392) -> (x .and. y?=w393:bool)
                n178 = case shown="True" w393 {
                  tunnel: [w397 w406] -> w395
                  tunnel: w394 -> [w397 w401]
                  frame False {
                  }
                  frame True {
                    n179 = local read "SOAK(m)"() -> (w398:dbl)
                    n180 = global read "Station References Global.vi" "Oven"() -> (w400:refnum<visa-resource-name>)
                    n181 = local read "TEMP"() -> (w405:dbl)
                    n182 = call "PM9 Set Temp and Wait.vi"("VISA"=w400, "Error In"=w401, "Accuracy +/-"=1.0, "Set Point"=w405, "RO(t)"=FALSE, "Min (-1 for cont.)"=w398, "close session(t)"=TRUE) -> ("session out"=→"ILabVIEW":refnum<k24>, "error out"=w406:errorcluster)  [unwired: 9 in, 2 out]
                  }
                }
              }
            }
          }
          frame #5 {
          }
          frame #6 {
            n183 = flat-sequence {
              tunnel: [w414] -> w408
              frame #0 {
                (unwired) FALSE
                # "Move The Gantry"
                n184 = local read "TX_PORT(t)"() -> (w413:bool)
                n185 = local read "GANTRY(t)"() -> (w412:bool)
                n186 = local read "ess_error"() -> (w410:errorcluster)
                n187 = And(x=w413, y=w412) -> (x .and. y?=w411:bool)
                n188 = case shown="True" w411 {
                  tunnel: w410 -> [w415 w422]
                  tunnel: [w415 w421] -> w414
                  frame False {
                  }
                  frame True {
                    w416 = u16 0 items=["Inches", "cm"] ("Zunits")
                    n189 = global read "Tetra_Globals.vi" "Gantry_Z"() -> (w418:dbl)
                    n190 = local read "TX_PORT"() -> (w423:i32)
                    n191 = global read "Station References Global.vi" "Gantry"() -> (w419:refnum<visa-resource-name>)
                    n192 = call "Gantry.vi"("COMPORT"=w419, "error in (no error)"=w422, "Antenna Select"=w423, "z ref"=21.0, "Write(reads antenna co-ords when off)"=TRUE, "z"=w418, "Zunits"=w416) -> ("error out"=w421:errorcluster)  [unwired: 12 in]
                  }
                }
              }
            }
            n193 = local write "ess_error"(w408) -> ()
          }
          frame #7 {
          }
          frame #8 {
            n194 = flat-sequence {
              tunnel: [w429] -> w426
              tunnel: w425 -> [w428]
              frame #0 {
                # "Program the Power Supply"
                n195 = local read "V_SUPPLY(t)"() -> (w427:bool)
                n196 = case shown="True" w427 {
                  tunnel: [w430 w432] -> w429
                  tunnel: w428 -> [w430 w431]
                  frame False {
                  }
                  frame True {
                    w435 = "PS1"  # SEL_PS
                    n197 = local read "V_SUPPLY"() -> (w434:dbl)
                    n198 = global read "Station References Global.vi" "PS1"() -> (w436:refnum<visa-resource-name>)
                    n199 = call "INST_PS_SET_VOLTAGE_LEVEL_4.0.0.vi"("Instrument Select (Output 1)"="1", "SEL_PS"=w435, "error in (no error)"=w431, "Voltage (0.0)"=w434, "VISA session"=w436) -> ("error out"=w432:errorcluster)  [unwired: 5 in, 1 out]
                  }
                }
              }
            }
          }
          frame #9 {
            n200 = call <vilib>:"High Resolution Relative Seconds.vi"() -> ("relative seconds"=w437:dbl)
          }
          frame #10 {
            n201 = flat-sequence {
              tunnel: [w449] -> w441
              tunnel: w440 -> [w447]
              frame #0 {
                # "Program the Settings"
                n202 = local read "MODE"() -> (w448:bool)
                n203 = case shown="True" w448 {
                  tunnel: [w462 w520] -> w449
                  tunnel: w447 -> [w461 w536]
                  tunnel: [w459 w530] -> w443
                  tunnel: [w458 w530] -> w444
                  tunnel: [w457 w529] -> w445
                  tunnel: [w450 i32[] [-1, -1, -1, -1] ("atten(code)ary (ro)")] -> w446
                  tunnel: [w451 w529] -> w442
                  frame False {
                    n204 = local read "ADAR_ATT(t)"() -> (w456:bool)
                    n205 = local read "comport"() -> (w452:refnum<visa-resource-name>)
                    n206 = case shown="True" w456 {
                      tunnel: w452 -> [w469 w477]
                      tunnel: [w470 w476] -> w465
                      tunnel: [w468 w471] -> w459
                      tunnel: w461 -> [w470 w473]
                      tunnel: [w469 w472] -> w460
                      frame False {
                        n207 = global read "Tetra_Globals.vi" "Atten0"() -> (w468:dbl)
                      }
                      frame True {
                        n208 = local read "ADAR ATT"() -> (w474:dbl)
                        n209 = call "Tetra_Atten.vi"("COMPORT"=w477, "error in (no error)"=w473, "TxAtten(num)"=0, "Atten(dB)"=w474) -> ("atten(value)"=w471:dbl, "comport"=w472:refnum<visa-resource-name>, "error out"=w476:errorcluster)  [unwired: 11 in, 2 out]
                      }
                    }
                    n210 = local read "EXT_ATT(t)"() -> (w455:bool)
                    n211 = case shown="True" w455 {
                      tunnel: [w481 w485] -> w467
                      tunnel: [w482 w490] -> w466
                      tunnel: w465 -> [w481 w494]
                      tunnel: [w479 w483] -> w457
                      tunnel: [w480 w484] -> w458
                      tunnel: w460 -> [w482 w491]
                      tunnel: [w478 w488] -> w450
                      frame False {
                        n212 = global read "Tetra_Globals.vi" "atten(code)ary (ro)"() -> (w478:i32[])
                        n213 = global read "Tetra_Globals.vi" "txatten-sel"() -> (w479:i32)
                        n214 = global read "Tetra_Globals.vi" "Atten1-3"() -> (w480:dbl)
                      }
                      frame True {
                        n215 = local read "TX_PORT"() -> (w492:i32)
                        n216 = local read "EXT_ATT"() -> (w493:dbl)
                        n217 = call "Port To Atten Map.vi"("Port"=w492, "error in"=w494) -> ("error out"=w495:errorcluster, "txatten-sel"=w483:i32)  [unwired: 8 in]
                        n218 = call "Tetra_Atten.vi"("COMPORT"=w491, "error in (no error)"=w495, "TxAtten(num)"=w483, "Atten(dB)"=w493) -> ("atten(value)"=w484:dbl, "comport"=w489:refnum<visa-resource-name>, "error out"=w486:errorcluster)  [unwired: 11 in, 2 out]
                        n219 = call "Tetra_Atten.vi"("COMPORT"=w489, "error in (no error)"=w486, "RO(t)"=TRUE) -> ("comport"=w490:refnum<visa-resource-name>, "atten(code)ary (ro)"=w488:i32[], "error out"=w485:errorcluster)  [unwired: 12 in, 2 out]
                      }
                    }
                    n220 = local read "TX_FILT(t)"() -> (w454:bool)
                    n221 = case shown="True" w454 {
                      tunnel: w467 -> [w498 w503]
                      tunnel: w466 -> [w497 w506]
                      tunnel: [w497 w505] -> w464
                      tunnel: [w498 w502] -> w463
                      tunnel: [w496 w500] -> w451
                      frame False {
                        n222 = global read "Tetra_Globals.vi" "TX_FILTER"() -> (w496:i32)
                      }
                      frame True {
                        w504 = 1 items=["RX", "TX"] ("RX/TX")
                        n223 = local read "TX_FILTER"() -> (w501:i32)
                        n224 = call "Tetra_Filt.vi"("COMPORT"=w506, "error in (no error)"=w503, "RO(t)"=FALSE, "RX/TX"=w504, "Filt(sel)"=w501) -> ("filt(num)"=w500:i32, "comport"=w505:refnum<visa-resource-name>, "error out"=w502:errorcluster)  [unwired: 12 in]
                      }
                    }
                    n225 = local read "TX_PORT(t)"() -> (w453:bool)
                    n226 = case shown="True" w453 {
                      tunnel: w464 -> [_ w512]
                      tunnel: w463 -> [w507 w511]
                      tunnel: [w507 w509] -> w462
                      frame False {
                      }
                      frame True {
                        w510 = 1 items=["RX", "TX"] ("TX/RX")
                        n227 = local read "TX_PORT"() -> (w508:i32)
                        n228 = global write "Tetra_Globals.vi" "TX_PORT"(w508) -> ()
                        n229 = call "Tetra_AntSel.vi"("COMPORT"=w512, "error in (no error)"=w511, "RX/TX"=w510, "ANT(num)"=w508) -> ("error out"=w509:errorcluster)  [unwired: 13 in, 2 out]
                      }
                    }
                  }
                  frame True {
                    w529 = -1 ("txatten-sel")
                    w530 = -1.0 ("atten(value)")
                    # "Program the Settings"
                    n230 = local read "RF_FREQ(t)"() -> (w515:bool)
                    n231 = local read "comport"() -> (w534:refnum<visa-resource-name>)
                    n232 = case shown="True" w515 {
                      tunnel: w534 -> [w553 w559]
                      tunnel: [w554 w556] -> w533
                      tunnel: w536 -> [w554 w560]
                      tunnel: [w553 w555] -> w532
                      frame False {
                      }
                      frame True {
                        w558 = u16 1 items=["MHz", "GHz"] ("Freq Units")
                        n233 = local read "RF_FREQ"() -> (w557:dbl)
                        n234 = call "Tetra_Set-Freq.vi"("COMPORT"=w559, "error in (no error)"=w560, "Freq"=w557, "Freq Units"=w558) -> ("comport"=w555:refnum<visa-resource-name>, "error out"=w556:errorcluster)  [unwired: 12 in, 2 out]
                      }
                    }
                    n235 = local read "TX_PORT(t)"() -> (w535:bool)
                    n236 = case shown="True" w535 {
                      tunnel: w532 -> [w561 w568]
                      tunnel: w533 -> [w562 w567]
                      tunnel: [w562 w565] -> w528
                      tunnel: [w561 w563] -> w527
                      frame False {
                      }
                      frame True {
                        w566 = 1 items=["RX", "TX"] ("TX/RX")
                        n237 = local read "TX_PORT"() -> (w564:i32)
                        n238 = global write "Tetra_Globals.vi" "TX_PORT"(w564) -> ()
                        n239 = call "Tetra_AntSel.vi"("COMPORT"=w568, "error in (no error)"=w567, "RX/TX"=w566, "ANT(num)"=w564) -> ("comport"=w563:refnum<visa-resource-name>, "error out"=w565:errorcluster)  [unwired: 13 in, 1 out]
                      }
                    }
                    n240 = local read "ADAR_ATT(t)"() -> (w517:bool)
                    n241 = local read "use-adar(t)"() -> (w525:bool)
                    n242 = And(x=w515, y=w517) -> (x .and. y?=w518:bool)
                    n243 = And(x=w517, y=w525) -> (x .and. y?=w526:bool)
                    n244 = Or(x=w518, y=w526) -> (x .or. y?=w519:bool)
                    n245 = case shown="True" w519 {
                      tunnel: w527 -> [w545 w552]
                      tunnel: w528 -> [w546 w551]
                      tunnel: [w546 w550] -> w522
                      tunnel: [w545 w547] -> w521
                      frame False {
                      }
                      frame True {
                        n246 = local read "ADAR ATT"() -> (w549:dbl)
                        n247 = call "Tetra_Atten.vi"("COMPORT"=w552, "error in (no error)"=w551, "TxAtten(num)"=0, "Atten(dB)"=w549) -> ("comport"=w547:refnum<visa-resource-name>, "error out"=w550:errorcluster)  [unwired: 11 in, 3 out]
                      }
                    }
                    n248 = local read "EXT_ATT(t)"() -> (w513:bool)
                    n249 = local read "use-psa(t)"() -> (w524:bool)
                    n250 = And(x=w515, y=w513) -> (x .and. y?=w514:bool)
                    n251 = And(x=w513, y=w524) -> (x .and. y?=w523:bool)
                    n252 = Or(x=w514, y=w523) -> (x .or. y?=w516:bool)
                    n253 = case shown="True" w516 {
                      tunnel: w521 -> [_ w544]
                      tunnel: w522 -> [w537 w541]
                      tunnel: [w537 w543] -> w520
                      frame False {
                      }
                      frame True {
                        n254 = global read "Tetra_Globals.vi" "TX_PORT"() -> (w539:i32)
                        n255 = local read "EXT_ATT"() -> (w542:dbl)
                        n256 = call "Port To Atten Map.vi"("Port"=w539, "error in"=w541) -> ("error out"=w540:errorcluster, "txatten-sel"=w538:i32)  [unwired: 8 in]
                        n257 = call "Tetra_Atten.vi"("COMPORT"=w544, "error in (no error)"=w540, "TxAtten(num)"=w538, "Atten(dB)"=w542) -> ("error out"=w543:errorcluster)  [unwired: 11 in, 4 out]
                      }
                    }
                  }
                }
                "adar-att(val)" <- w443
                "ext-atten(val)" <- w444
                "txatten-sel" <- w445
                "atten(code)ary (ro)" <- w446
                "filt(num)" <- w442
                n258 = global write "Tetra_Globals.vi" "Atten0"(w443) -> ()
                n259 = global write "Tetra_Globals.vi" "Atten1-3"(w444) -> ()
                n260 = global write "Tetra_Globals.vi" "atten(code)ary (ro)"(w446) -> ()
                n261 = global write "Tetra_Globals.vi" "txatten-sel"(w445) -> ()
                n262 = global write "Tetra_Globals.vi" "TX_FILTER"(w442) -> ()
              }
            }
          }
          frame #11 {
            n263 = call <vilib>:"High Resolution Relative Seconds.vi"() -> ("relative seconds"=w571:dbl)
            n264 = Subtract(x=w571, y=w570) -> (x-y=→"x-y":dbl)
          }
          frame #12 {
            n265 = flat-sequence {
              tunnel: [w581] -> w574
              tunnel: w573 -> [w580]
              frame #0 {
                # "Get the DC Currents from Power Sup"
                n266 = local read "V_SUPPLY(t)"() -> (w577:bool)
                n267 = local read "TEMP(t)"() -> (w576:bool)
                n268 = local read "MEAS_PS"() -> (w579:bool)
                n269 = Or(x=w577, y=w576) -> (x .or. y?=w575:bool)
                n270 = Or(x=w575, y=w579) -> (x .or. y?=w578:bool)
                n271 = case shown="True" w578 {
                  tunnel: [dbl[] [-1.0, -1.0] w588] -> w582
                  tunnel: [w584 w591] -> w581
                  tunnel: w580 -> [w584 w592]
                  frame False {
                  }
                  frame True {
                    w595 = 0 items=["Current", "Voltage"] ("Measurement Type (1: Voltage)")
                    w594 = "PS1"  # SEL_PS
                    n272 = global read "Station References Global.vi" "PS1"() -> (w593:refnum<visa-resource-name>)
                    n273 = call "PS_MEASURE_V-I_Ary.vi"("VISA resource name"=w593, "SEL_PS"=w594, "error in (no error)"=w592, "Array 2"=bool[] [TRUE, FALSE, FALSE, FALSE], "Measurement Type (1: Voltage)"=w595) -> ("Array"=w589:dbl[], "error out"=w591:errorcluster)  [unwired: 8 in, 1 out]
                    n274 = local read "V_SUPPLY"() -> (w587:dbl)
                    n275 = Index Array(array=w589) -> (element=w585:dbl)  [unwired: 1 in]
                    n276 = Multiply(x=w585, y=w587) -> (x*y=w586:dbl)
                    n277 = Build Array(w585, w586) -> (w588:dbl[])
                  }
                }
                "ps_meas(i)(w)" <- w582
              }
            }
          }
          frame #13 {
          }
          frame #14 {
            n278 = flat-sequence {
              tunnel: w602 -> [w605]
              tunnel: [w603] -> w601
              tunnel: w601 -> [w614]
              tunnel: [w612] -> w600
              tunnel: w600 -> [w626]
              tunnel: [w625] -> w599
              tunnel: w599 -> [w632]
              tunnel: [w631] -> w598
              tunnel: w598 -> [w664]
              tunnel: [w649] -> w597
              frame #0 {
                # "Set The REF power"
                n279 = local read "REF_PWR(t)"() -> (w604:bool)
                n280 = case shown="True" w604 {
                  tunnel: w605 -> [w606 w610]
                  tunnel: [w606 w611] -> w603
                  frame False {
                  }
                  frame True {
                    (unwired) FALSE ("RO(T)")
                    w607 = 1 ("CH")
                    n281 = local read "REF_POW"() -> (w609:dbl)
                    n282 = global read "Station References Global.vi" "PNA"() -> (w608:refnum<visa-resource-name>)
                    n283 = call "Configure Power.vi"("VISA resource name"=w608, "Channel (1)"=w607, "Port (1)"=w607, "error in (no error)"=w610, "Power Level (0 dBm)"=w609) -> ("error out"=w611:errorcluster)  [unwired: 9 in, 1 out]
                  }
                }
              }
              frame #1 {
                # "Set The REF Fixed Freq"
                n284 = local read "RF_FREQ(t)"() -> (w613:bool)
                n285 = case shown="True" w613 {
                  tunnel: w614 -> [w615 w623]
                  tunnel: [w615 w619] -> w612
                  frame False {
                  }
                  frame True {
                    w616 = 0 items=["Normal", "SMC"] ("MODE")
                    w617 = i64 1000000000 items=["GHz"=1000000000, "MHZ"=1000000] ("Units")
                    n286 = global read "Station References Global.vi" "PNA"() -> (w624:refnum<visa-resource-name>)
                    n287 = local read "f_ref"() -> (w620:dbl)
                    n288 = call "PNA-L_SET-CWFREQ.vi"("Session In"=w624, "error in"=w623, "MODE"=w616, "FREQ"=w620, "Units"=w617, "RO(T)"=FALSE, "CH"=1, "Source"=1) -> ("error out"=w619:errorcluster)  [unwired: 9 in, 2 out]
                  }
                }
              }
              frame #2 {
                w628 = 3 items=["HOLD", "CONT", "GROUP", "SINGLE"]  # Mode
                w627 = 1  # Channel
                # "Take the Sweep with The PNA"
                n289 = global read "Station References Global.vi" "PNA"() -> (w629:refnum<visa-resource-name>)
                n290 = call "PNA_SWEEP MODE.vi"("Mode"=w628, "Channel"=w627, "error in (no error)"=w626, "VISA resource name"=w629) -> ("error out"=w625:errorcluster)  [unwired: 6 in, 1 out]
              }
              frame #3 {
                # "Meas S11 on the PNA"
                n291 = local read "MEAS_S11"() -> (w633:bool)
                n292 = case shown="True" w633 {
                  tunnel: w632 -> [w635 _]
                  tunnel: [w635 w642] -> w631
                  tunnel: [-1.0 w641] -> w630
                  frame False {
                  }
                  frame True {
                    w637 = 1 ("Channel (1)")
                    n293 = global read "Station References Global.vi" "PNA"() -> (w638:refnum<visa-resource-name>)
                    n294 = call "Select Measurement.vi"("Measurement Name (CH1_S11_1)"="CH1_S11_1", "Channel (1)"=w637, "VISA resource name"=w638) -> ("error out"=w639:errorcluster, "VISA resource name out"=w640:refnum<visa-resource-name>)  [unwired: 7 in]
                    n295 = call "PNA-L_MKR_RageATE.vi"("VISA resource name"=w640, "Channel (1)"=w637, "Trace (1)"=w637, "Marker (1)"=w637, "error in (no error)"=w639) -> ("Y Real Value"=w641:dbl, "error out"=w642:errorcluster)  [unwired: 6 in, 3 out]
                  }
                }
                "s11" <- w630
              }
              frame #4 {
                n296 = global read "Station References Global.vi" "Spectrum Analyzer Present?"() -> (w662:bool)
                n297 = case shown="True" w662 {
                  tunnel: w664 -> [w724 w744]
                  tunnel: [dbl[] [-1.0, -1.0] ("Mark Values") w734] -> w663
                  tunnel: [w724 w736] -> w661
                  tunnel: [w723 w728] -> w655
                  tunnel: [w723 w727] -> w645
                  frame False {
                    w723 = -1.0 ("Ampl_corr")
                  }
                  frame True {
                    w735 = u16 2 items=["Hz", "MHz", "GHz"] ("Freq Units")
                    w740 = TRUE ("AVG Restart (T)")
                    w741 = 1 items=["Clear Write", "Average", "Maximum Hold", "Minimum Hold"] ("Trace Type (0: Clear Write)")
                    n298 = global read "Station References Global.vi" "Spectrum Analyzer"() -> (w745:refnum<visa-resource-name>)
                    n299 = local read "RF_FREQ"() -> (w738:dbl)
                    n300 = call "SA_SET_CF.vi"("Send OPC? (T)"=TRUE, "READ ONLY (T)"=FALSE, "error in"=w744, "Freq Units"=w735, "SET CF ()"=w738, "Session In"=w745) -> ("error out"=w730:errorcluster, "Session Out"=w731:refnum<visa-resource-name>)  [unwired: 3 in, 1 out]
                    n301 = local read "AVG"() -> (w739:i32)
                    n302 = local read "out_cal_ampl"() -> (w729:dbl)
                    n303 = call "SA_AVG.vi"("Session In"=w731, "AVG Count"=w739, "error in"=w730, "Trace Type (0: Clear Write)"=w741, "AVG Restart (T)"=w740, "Send OPC? (T)"=w740) -> ("Session Out"=w732:refnum<visa-resource-name>, "error out"=w733:errorcluster)  [unwired: 8 in]
                    n304 = local read "fsl_corr_dB"() -> (w726:dbl)
                    n305 = call "SA_GET_MARKER.vi"("offset"=w729, "Set MKR Freq ()"=w738, "Use PK Search (T)"=TRUE, "error in"=w733, "Session In"=w732) -> ("error out"=w736:errorcluster, "Ampl_corr"=w728:dbl, "Mark Values"=w734:dbl[])  [unwired: 3 in, 1 out]
                    n306 = Add(x=w728, y=w726) -> (x+y=w727:dbl)
                  }
                }
                "exa_mkr" <- w663
                "Ampl_corr" <- w655
                "fsl_ampl_corr" <- w645
                n307 = global read "Station References Global.vi" "Spectrum Analyzer Present?"() -> (w658:bool)
                n308 = local read "h2(t)"() -> (w657:bool)
                n309 = And(x=w658, y=w657) -> (x .and. y?=w659:bool)
                n310 = case shown="True" w659 {
                  tunnel: w661 -> [w695 w721]
                  tunnel: [dbl[] [-1.0, -1.0] ("Mark Values") w706] -> w660
                  tunnel: [w695 w709] -> w650
                  tunnel: [w694 w703] -> w656
                  tunnel: [w694 w698] -> w654
                  tunnel: [w694 w697] -> w644
                  frame False {
                    w694 = -1.0
                    n311 = local write "h2_cal_ampl"(w694) -> ()
                    n312 = local write "h2_cal freq"(w694) -> ()
                  }
                  frame True {
                    w708 = u16 2 items=["Hz", "MHz", "GHz"] ("Freq Units")
                    w715 = TRUE ("AVG Restart (T)")
                    w716 = 1 items=["Clear Write", "Average", "Maximum Hold", "Minimum Hold"] ("Trace Type (0: Clear Write)")
                    n313 = global read "Station References Global.vi" "Spectrum Analyzer"() -> (w722:refnum<visa-resource-name>)
                    n314 = local read "H2_FREQ"() -> (w711:dbl)
                    n315 = call "GLOBAL CENTER FREQ.vi"("Send OPC? (T)"=TRUE, "READ ONLY (T)"=FALSE, "error in"=w721, "Freq Units"=w708, "SET CF ()"=w711, "Session In"=w722) -> ("error out"=w717:errorcluster, "Session Out"=w718:refnum<visa-resource-name>)  [unwired: 3 in, 1 out]
                    n316 = local read "AVG"() -> (w714:i32)
                    n317 = local read "h2_cal_ampl"() -> (w700:dbl)
                    n318 = call "AVG_TRACE.vi"("Session In"=w718, "AVG Count"=w714, "error in"=w717, "Trace Type (0: Clear Write)"=w716, "AVG Restart (T)"=w715, "Send OPC? (T)"=w715) -> ("Session Out"=w712:refnum<visa-resource-name>, "error out"=w713:errorcluster)  [unwired: 8 in]
                    n319 = local read "fsl_corr_dB"() -> (w699:dbl)
                    n320 = local read "exa_mkr"() -> (w707:dbl[])
                    n321 = call "GET_MARKER.vi"("offset"=w700, "Set MKR Freq (MHz)"=w711, "Use PK Search (T)"=TRUE, "error in"=w713, "Session In"=w712) -> ("error out"=w709:errorcluster, "Ampl_corr"=w698:dbl, "Mark Values"=w706:dbl[])  [unwired: 3 in, 1 out]
                    n322 = Add(x=w698, y=w699) -> (x+y=w697:dbl)
                    n323 = Index Array(array=w706, index=1) -> (element=w702:dbl)
                    n324 = Index Array(array=w707, index=1) -> (element=w701:dbl)
                    n325 = Subtract(x=w702, y=w701) -> (x-y=w703:dbl)
                  }
                }
                "h2_mkr" <- w660
                "h2_dbc" <- w656
                "h2_corr" <- w654
                "h2_fsl_corr" <- w644
                n326 = global read "Station References Global.vi" "Spectrum Analyzer Present?"() -> (w647:bool)
                n327 = local read "hx(t)"() -> (w648:bool)
                n328 = And(x=w647, y=w648) -> (x .and. y?=w646:bool)
                n329 = case shown="True" w646 {
                  tunnel: w650 -> [w666 w692]
                  tunnel: [dbl[] [-1.0, -1.0] ("Mark Values") w677] -> w652
                  tunnel: [w666 w680] -> w649
                  tunnel: [w665 w674] -> w651
                  tunnel: [w665 w670] -> w653
                  tunnel: [w665 w669] -> w643
                  frame False {
                    w665 = -1.0
                    n330 = local write "hx_cal freq"(w665) -> ()
                    n331 = local write "hx_cal_ampl"(w665) -> ()
                  }
                  frame True {
                    w679 = u16 2 items=["Hz", "MHz", "GHz"] ("Freq Units")
                    w686 = TRUE ("AVG Restart (T)")
                    w687 = 1 items=["Clear Write", "Average", "Maximum Hold", "Minimum Hold"] ("Trace Type (0: Clear Write)")
                    n332 = global read "Station References Global.vi" "Spectrum Analyzer"() -> (w693:refnum<visa-resource-name>)
                    n333 = local read "Hx_FREQ"() -> (w682:dbl)
                    n334 = call "GLOBAL CENTER FREQ.vi"("Send OPC? (T)"=TRUE, "READ ONLY (T)"=FALSE, "error in"=w692, "Freq Units"=w679, "SET CF ()"=w682, "Session In"=w693) -> ("error out"=w688:errorcluster, "Session Out"=w689:refnum<visa-resource-name>)  [unwired: 3 in, 1 out]
                    n335 = local read "AVG"() -> (w685:i32)
                    n336 = local read "hx_cal_ampl"() -> (w672:dbl)
                    n337 = call "AVG_TRACE.vi"("Session In"=w689, "AVG Count"=w685, "error in"=w688, "Trace Type (0: Clear Write)"=w687, "AVG Restart (T)"=w686, "Send OPC? (T)"=w686) -> ("Session Out"=w683:refnum<visa-resource-name>, "error out"=w684:errorcluster)  [unwired: 8 in]
                    n338 = local read "fsl_corr_dB"() -> (w668:dbl)
                    n339 = local read "exa_mkr"() -> (w678:dbl[])
                    n340 = call "GET_MARKER.vi"("offset"=w672, "Set MKR Freq (MHz)"=w682, "Use PK Search (T)"=TRUE, "error in"=w684, "Session In"=w683) -> ("error out"=w680:errorcluster, "Ampl_corr"=w670:dbl, "Mark Values"=w677:dbl[])  [unwired: 3 in, 1 out]
                    n341 = Add(x=w670, y=w668) -> (x+y=w669:dbl)
                    n342 = Index Array(array=w677, index=1) -> (element=w673:dbl)
                    n343 = Index Array(array=w678, index=1) -> (element=w671:dbl)
                    n344 = Subtract(x=w673, y=w671) -> (x-y=w674:dbl)
                  }
                }
                "hx_dbc" <- w651
                "hx_mkr" <- w652
                "hx_corr" <- w653
                "hx_fsl_corr" <- w643
              }
            }
          }
          frame #15 {
            # "Get the chip stuff..."
            n345 = flat-sequence {
              tunnel: w748 -> [w753]
              tunnel: [w752] -> w750
              tunnel: w750 -> [w770]
              tunnel: [w771] -> w749
              tunnel: w749 -> [w803]
              tunnel: [w805] -> w747
              tunnel: [w824] -> w746
              tunnel: w747 -> [w825]
              frame #0 {
                # "Get the Power detector"
                n346 = local read "GET_DETECT"() -> (w751:bool)
                n347 = case shown="True" w751 {
                  tunnel: [-1.0 w761] -> w754
                  tunnel: w753 -> [w755 w759]
                  tunnel: [w755 w760] -> w752
                  frame False {
                  }
                  frame True {
                    n348 = local read "comport"() -> (w757:refnum<visa-resource-name>)
                    n349 = local read "TX_PORT"() -> (w758:i32)
                    n350 = call "TX-ADAR-DETECT.vi"("COMPORT"=w757, "error in (no error)"=w759, "Ant_Sel"=w758) -> ("adc read"=w761:dbl, "error out"=w760:errorcluster)  [unwired: 9 in, 2 out]
                  }
                }
                "detect" <- w754
              }
              frame #1 {
                n351 = local read "MEAS_DCMON"() -> (w766:bool)
                n352 = local read "TEMP(t)"() -> (w767:bool)
                n353 = local read "MEAS_DCMON"() -> (w768:bool)
                n354 = Or(x=w767, y=w766) -> (x .or. y?=w765:bool)
                n355 = local read "V_SUPPLY(t)"() -> (w764:bool)
                n356 = Or(x=w765, y=w768) -> (x .or. y?=w769:bool)
                n357 = Or(x=w769, y=w764) -> (x .or. y?=w763:bool)
                n358 = case shown="True" w763 {
                  tunnel: [w782 w800] -> w772
                  tunnel: [w782 w799] -> w773
                  tunnel: [w780 w798] -> w771
                  tunnel: [w783 w797] -> w774
                  tunnel: w770 -> [w780 w792]
                  tunnel: [FALSE w789] -> w762
                  frame False {
                    n359 = global read "Tetra_Globals.vi" "RevC(t)"() -> (w778:bool)
                    n360 = Select(t=11, s=w778, f=10) -> (s? t:f=w775:i32)
                    n361 = for {
                      N: 6 -> [_]
                      tunnel: [-1.0] -> w782 mode=indexing
                    }
                    n362 = for {
                      N: w775 -> [_]
                      tunnel: [-1.0] -> w783 mode=indexing
                    }
                  }
                  frame True {
                    # "need to add rdv screen"
                    n363 = local read "comport"() -> (w791:refnum<visa-resource-name>)
                    n364 = local read "support_path"() -> (w786:path)
                    n365 = call "Tetra_Read UCD.vi"("COMPORT"=w791, "error in (no error)"=w792) -> ("rdv"=w797:dbl[], "comport"=w795:refnum<visa-resource-name>, "error out"=w796:errorcluster)  [unwired: 11 in]
                    n366 = local read "RevC(t)"() -> (w787:bool)
                    n367 = call "Time Delay"("error in (no error)"=w796, "Delay Time (s)"=0.01) -> ("error out"=w794:errorcluster)  [unwired: 9 in]
                    n368 = call "Tetra_Read Imon.vi"("COMPORT"=w795, "ini limits directory (if blank will skip)"=w786, "rev_c(t)"=w787, "error in (no error)"=w794, "Meas_Limits"=TRUE) -> ("rdiv(i)"=w800:dbl[], "rdiv(v)"=w799:dbl[], "Fail?(t)"=w790:bool, "error out"=w798:errorcluster)  [unwired: 9 in, 2 out]
                    n369 = Not(x=w790) -> (.not. x?=w789:bool)
                  }
                }
                "rdiv(i)" <- w772
                "rdiv(v)" <- w773
                "rdv" <- w774
                "imon_pass?(t)" <- w762
              }
              frame #2 {
                n370 = local read "CHIP_TEMP(t)"() -> (w802:bool)
                n371 = case shown="True" w802 {
                  tunnel: [w807 w809] -> w805
                  tunnel: [dbl[] [-1.0, -1.0, -1.0, -1.0, -1.0, -1.0] ("Deg") w810] -> w801
                  tunnel: w803 -> [w807 w818]
                  tunnel: ["-1" ("temp 0x") w817] -> w804
                  frame False {
                  }
                  frame True {
                    n372 = local read "comport"() -> (w816:refnum<visa-resource-name>)
                    n373 = call "TX-ADAR-TEMP.vi"("COMPORT"=w816, "error in (no error)"=w818) -> ("temp 0x"=w817:string, "comport"=w815:refnum<visa-resource-name>, "temp(c)"=w812:dbl, "error out"=w814:errorcluster)  [unwired: 10 in]
                    n374 = call "ReadTempSense.vi"("COMPORT"=w815, "error in (no error)"=w814) -> ("temp(c)"=w813:dbl[], "error out"=w809:errorcluster)  [unwired: 10 in, 2 out]
                    n375 = Insert Into Array(array=w813, index=0, new element=w812) -> (w810:dbl[])
                  }
                }
                "temp_data" <- w801
                "temp 0x" <- w804
              }
              frame #3 {
                n376 = local read "FiltRead"() -> (w819:bool)
                n377 = local read "MODE"() -> (w823:bool)
                n378 = Or(x=w823, y=w819) -> (x .or. y?=w820:bool)
                n379 = case shown="True" w820 {
                  tunnel: w825 -> [w827 w838]
                  tunnel: [w827 w835] -> w824
                  tunnel: [w826 w832] -> w822
                  tunnel: [w826 w828] -> w821
                  frame False {
                    w826 = -1 ("bpf")
                  }
                  frame True {
                    w830 = 1 items=["RX", "TX"] ("RX/TX")
                    w840 = 1 items=["RX", "TX"] ("RX/TX")
                    n380 = local read "comport"() -> (w837:refnum<visa-resource-name>)
                    n381 = call "Tetra_Filt.vi"("COMPORT"=w837, "error in (no error)"=w838, "RO(t)"=TRUE, "RX/TX"=w840) -> ("filt(num)"=w828:i32, "comport"=w842:refnum<visa-resource-name>, "error out"=w841:errorcluster)  [unwired: 13 in]
                    n382 = call "Tetra_Atten.vi"("COMPORT"=w842, "error in (no error)"=w841, "RO(t)"=TRUE) -> ("comport"=w833:refnum<visa-resource-name>, "atten(code)ary (ro)"=w836:i32[], "error out"=w834:errorcluster)  [unwired: 12 in, 2 out]
                    n383 = global write "Tetra_Globals.vi" "atten(code)ary (ro)"(w836) -> ()
                    n384 = local write "atten(code)ary (ro)"(w836) -> ()
                    n385 = call "Tetra_BPF.vi"("COMPORT"=w833, "error in (no error)"=w834, "RO(t)"=TRUE, "RX/TX"=w830) -> ("bpf"=w832:i32, "error out"=w835:errorcluster)  [unwired: 13 in, 1 out]
                  }
                }
                "bpf" <- w822
                n386 = local write "filt(num)"(w821) -> ()
                n387 = global write "Tetra_Globals.vi" "TX_FILTER"(w821) -> ()
              }
            }
          }
          frame #16 {
          }
          frame #17 {
            n388 = flat-sequence {
              tunnel: [w851] -> w845
              tunnel: w844 -> [w846]
              frame #0 {
                n389 = local read "PLATE_TEMP(t)"() -> (w849:bool)
                n390 = global read "Station References Global.vi" "Oven Present?"() -> (w847:bool)
                n391 = And(x=w849, y=w847) -> (x .and. y?=w848:bool)
                n392 = case shown="True" w848 {
                  tunnel: [w853 w857] -> w851
                  tunnel: [sgl[] [-1.0, -1.0] w855] -> w850
                  tunnel: w846 -> [w853 w856]
                  frame False {
                  }
                  frame True {
                    n393 = for {
                      N: 3 -> [_]
                      tunnel: [w861] -> w855
                      shift-right: [w858] -> w857
                      shift-left: w856 -> [w863]
                      stop <- w858 continue-if-true
                      w862 = u16 1 items=["SENSOR 1", "SENSOR 2"] ("Sensor")
                      w868 = u16 0 items=["SENSOR 1", "SENSOR 2"] ("Sensor")
                      n394 = global read "Station References Global.vi" "Oven"() -> (w870:refnum<visa-resource-name>)
                      n395 = call "PM9_TCP_READ-TEMP.vi"("VISA"=w870, "error in (no error)"=w863, "Sensor"=w868, "Close tcp(t)"=FALSE) -> ("Value"=w860:sgl, "visa out"=w866:refnum<visa-resource-name>, "connection ID out"=w865:refnum<k5>, "error out"=w867:errorcluster)  [unwired: 8 in]
                      n396 = call "PM9_TCP_READ-TEMP.vi"("VISA"=w866, "connection ID"=w865, "error in (no error)"=w867, "Sensor"=w862, "Close tcp(t)"=TRUE) -> ("Value"=w859:sgl, "error out"=w858:errorcluster)  [unwired: 7 in, 2 out]
                      n397 = Build Array(w860, w859) -> (w861:sgl[])
                    }
                  }
                }
                "plate_temp" <- w850
              }
            }
          }
          frame #18 {
            n398 = flat-sequence {
              tunnel: [w873] -> w871
              frame #0 {
                w874 = TRUE ("Close Serial")
                n399 = local read "ess_error"() -> (w879:errorcluster)
                n400 = global read "Station References Global.vi" "Gantry"() -> (w877:refnum<visa-resource-name>)
                n401 = local read "FH_NOT(T)"() -> (w876:bool)
                n402 = call "WAM_ESS.vi"("VISA resource name"=w877, "error in (no error)"=w879, "Open Serial"=w874, "Test Running (T)"=w874, "Close Serial"=w874) -> ("FH_NOT(T)"=w875:bool, "VISA resource name out"=w878:refnum<visa-resource-name>, "error out"=w880:errorcluster)  [unwired: 7 in, 1 out]
                n403 = And(x=w876, y=w875) -> (x .and. y?=w873:bool)
                "no_fault" <- w873
                n404 = case shown="False" w873 {
                  tunnel: w878 -> [w889 _]
                  tunnel: w880 -> [w888 w895]
                  tunnel: [w887 w895] -> w881
                  frame False {
                    w885 = u16 1 items=["Disable Driver", "Enable Driver", "Read Driver Status"] ("Driver-Func")
                    w886 = TRUE ("Close Serial")
                    n405 = call "Prompt User for Input"("error in (no error)"=w888) -> ("OK"=w884:bool, "error out"=w883:errorcluster)  [unwired: 17 in]
                    n406 = case shown="False" w884 {
                      selector: w884 -> [w891 _]
                      tunnel: w883 -> [w893 w894]
                      tunnel: [w892 w894] -> w882
                      frame False {
                        n407 = invoke class="VI" method="Abort VI"(error in=w893) -> (error out=w892:errorcluster)  [unwired: 2 in, 2 out]
                        n408 = Not(x=w891) -> (.not. x?=w890:bool)
                        n409 = local write "STOP(T)"(w890) -> ()
                        n410 = global write "Sequence Globals.vi" "Stop Testing"(w890) -> ()
                      }
                      frame True {
                      }
                    }
                    n411 = call "Gantry_Driver.vi"("VISA resource name"=w889, "error in (no error)"=w882, "Open Serial"=w886, "Driver-Func"=w885, "Close Serial"=w886) -> ("error out"=w887:errorcluster)  [unwired: 11 in, 3 out]
                  }
                  frame True {
                  }
                }
                n412 = local write "ess_error"(w881) -> ()
              }
            }
          }
          frame #19 {
            # "Insert the output numeric array data"
            n413 = Unbundle By Name(w898) -> ("status"=w897:bool)
            n414 = local read "relative seconds"() -> (w935:dbl)
            n415 = local read "atten(code)ary (ro)"() -> (w911:i32[])
            n416 = global read "Sequence Globals.vi" "Current Iteration"() -> (w934:i32)
            n417 = local read "horn_Ampl Out"() -> (w899:dbl)
            n418 = local read "ps_meas(i)(w)"() -> (w930:dbl[])
            n419 = local read "fsl_ampl_corr"() -> (w902:dbl)
            n420 = local read "ext-atten(val)"() -> (w928:dbl)
            n421 = local read "out_cal_ampl"() -> (w919:dbl)
            n422 = call <vilib>:"High Resolution Relative Seconds.vi"() -> ("relative seconds"=w936:dbl)
            "iteration time(s)" <- w936
            n423 = local read "adar-att(val)"() -> (w923:dbl)
            n424 = local read "h2_cal_ampl"() -> (w914:dbl)
            n425 = local read "hx_cal_ampl"() -> (w904:dbl)
            n426 = local read "out_cal freq"() -> (w918:dbl)
            n427 = local read "plate_temp"() -> (w925:sgl[])
            n428 = local read "temp_data"() -> (w924:dbl[])
            n429 = local read "fsl_corr_dB"() -> (w901:dbl)
            n430 = local read "h2_cal freq"() -> (w913:dbl)
            n431 = local read "hx_cal freq"() -> (w903:dbl)
            n432 = local read "Ampl_corr"() -> (w917:dbl)
            n433 = local read "filt(num)"() -> (w929:i32)
            n434 = local read "exa_mkr"() -> (w927:dbl[])
            n435 = local read "h2_mkr"() -> (w916:dbl[])
            n436 = local read "h2_dbc"() -> (w920:dbl)
            n437 = local read "h2_corr"() -> (w912:dbl)
            n438 = local read "hx_mkr"() -> (w907:dbl[])
            n439 = local read "hx_corr"() -> (w906:dbl)
            n440 = local read "hx_dbc"() -> (w905:dbl)
            n441 = Subtract(x=w936, y=w935) -> (x-y=w921:dbl)
            n442 = local read "rdiv(v)"() -> (w932:dbl[])
            n443 = local read "fsl(dB)"() -> (w900:dbl)
            n444 = local read "detect"() -> (w926:dbl)
            n445 = local read "rdiv(i)"() -> (w931:dbl[])
            n446 = local read "f_ref"() -> (w915:dbl)
            n447 = local read "rdv"() -> (w933:dbl[])
            n448 = local read "s11"() -> (w922:dbl)
            n449 = local read "bpf"() -> (w910:i32)
            n450 = Build Array (concatenate)(w930, w927, w917, w902, w922, w915, w916, w912, w920, w907, w906, w905, w926, w929, w910, w923, w928, w911, w933, w932, w931, w924, w925, w921, w934, w919, w918, w914, w913, w904, w903, w901, w900, w899) -> (w909:dbl[])
            n451 = for {
              tunnel: w909 -> [w940] mode=indexing
              tunnel: [w938] -> w908 mode=indexing
              n452 = Format Into String(format string="%#.3f", initial string="", w940) -> (resulting string=w938:string)  [unwired: 1 in, 1 out]
            }
            n453 = Not(x=w897) -> (.not. x?=w896:bool)
          }
        }
        n454 = Greater Than 0?(x=w41) -> (x > 0?=→"fault?(t)":bool)
        n455 = And(x=w42, y=w38) -> (x .and. y?=w39:bool)
      }
    }
    frame #2 {
      n456 = flat-sequence {
        tunnel: [w964] -> w954
        tunnel: [w963] -> w953
        tunnel: w954 -> [w968]
        tunnel: w953 -> [w965]
        tunnel: [w1025] -> w952
        tunnel: [w1021] -> w944
        frame #0 {
          # "Flag rows to report"
          n457 = local read "EXT_ATT"() -> (w964:dbl)
          n458 = local read "fsl_ampl_corr"() -> (w963:dbl)
        }
        frame #1 {
          # "Store tx data for reatreival to calc  flatness\nThis is based on 2 \"bands\"of 20-25, 25-*40 GHz"
          n459 = Current VI's Path() -> (path=w972:path)
          n460 = Multiply(x=w968, y=1000.0) -> (x*y=w967:dbl)
          n461 = Strip Path(path=w972) -> (stripped path=w969:path)  [unwired: 1 out]
          n462 = Build Path(base path=w969, name or relative path=path "txatten.txt" ("file path (dialog if empty)")) -> (appended path=w971:path)
          n463 = Build Array(w968, w965) -> (w973:dbl[])
          n464 = case shown="500.." w967 {
            tunnel: w971 -> [w981 w997]
            tunnel: w973 -> [w978 w988]
            frame 0, Default {
              n465 = Index Array(array=w978, index=1) -> (element=→"att_ref":dbl)
              n466 = local read "ADAR_ATT(t)"() -> (w974:bool)
              n467 = local read "TX_PORT(t)"() -> (w980:bool)
              n468 = Or(x=w974, y=w980) -> (x .or. y?=w975:bool)
              n469 = Not(x=w975) -> (.not. x?=w979:bool)
              n470 = call-poly <vilib>:"Write Delimited Spreadsheet.vi"("file path (dialog if empty)"=w981, "1D data"=w978, "append to file? (new file:F)"=w979) -> ()  [unwired: 11 in, 2 out]
            }
            frame 500.. {
              n471 = Index Array(array=w988, index #2=1 ("index")) -> (element #1=w984:dbl, element #2=w982:dbl)  [unwired: 1 in]
              n472 = call-poly <vilib>:"Write Delimited Spreadsheet.vi"("file path (dialog if empty)"=w997, "1D data"=w988, "append to file? (new file:F)"=TRUE) -> ("new file path (Not A Path if cancelled)"=w995:path, "error out"=w994:errorcluster)  [unwired: 11 in]
              n473 = flat-sequence {
                tunnel: [w1000] -> w996
                tunnel: w995 -> [w1002]
                tunnel: w994 -> [w1001]
                tunnel: [w999] -> w992
                tunnel: [w998] -> w990
                tunnel: w996 -> [w1016]
                tunnel: [w1015] -> w993
                tunnel: w992 -> [w1015]
                tunnel: [w1014] -> _
                tunnel: [w1013] -> w991
                tunnel: w990 -> [w1013]
                tunnel: w993 -> [w1020]
                tunnel: w988 -> [w1019]
                tunnel: w991 -> [w1018]
                frame #0 {
                  n474 = call-poly <vilib>:"Read Delimited Spreadsheet.vi"("file path (dialog if empty)"=w1002, "error in (no error)"=w1001) -> ("new file path (Not A Path if cancelled)"=w999:path, "all rows"=w1000:dbl[][], "error out"=w998:errorcluster)  [unwired: 8 in, 3 out]
                }
                frame #1 {
                  n475 = Index Array(array=w1016, index (col) #1=0 ("disabled index (col)"), index (col) #2=1 ("index (col)")) -> (element #1=w1012:dbl[], element #2=w1011:dbl[])  [unwired: 2 in]
                  n476 = Index Array(array=w1012) -> (element #1=w1008:dbl, element #2=w1007:dbl)  [unwired: 2 in]
                  n477 = Index Array(array=w1011) -> (element #1=w1006:dbl, element #2=w1005:dbl)  [unwired: 2 in]
                  n478 = Subtract(x=w1007, y=w1008) -> (x-y=w1003:dbl)
                  n479 = Subtract(x=w1006, y=w1005) -> (x-y=w1004:dbl)
                  n480 = Subtract(x=w1004, y=w1003) -> (x-y=w1014:dbl)
                  "att_dnl" <- w1014
                }
                frame #2 {
                  # "open a new file"
                  n481 = call-poly <vilib>:"Write Delimited Spreadsheet.vi"("file path (dialog if empty)"=w1020, "1D data"=w1019, "append to file? (new file:F)"=FALSE, "error in (no error)"=w1018) -> ()  [unwired: 10 in, 2 out]
                }
              }
              n482 = local read "att_ref"() -> (w983:dbl)
              n483 = Subtract(x=w983, y=w982) -> (x-y=w985:dbl)
              n484 = Subtract(x=w985, y=w984) -> (x-y=→"att_inl":dbl)
            }
          }
        }
        frame #2 {
          n485 = local read "RF_FREQ"() -> (w1024:dbl)
          n486 = local read "EXT_ATT"() -> (w1026:dbl)
          n487 = local read "att_dnl"() -> (w1023:dbl)
          n488 = call "PSA-Mask.vi"("Freq(GHZ)"=w1024, "Mask Offset dB"=0.25, "Error (dBin)"=w1023, "Att"=w1026) -> ("parsed result"=w1025:string[], "Pass(t)"=w1021:bool)  [unwired: 5 in, 1 out]
        }
      }
      n489 = flat-sequence {
        tunnel: [w1047] -> w958
        tunnel: [w1041] -> w957
        tunnel: [w1032] -> w955
        tunnel: [w1031] -> w948
        tunnel: [w1030] -> w947
        tunnel: [w1029] -> w946
        frame #0 {
          # "SPEC LIMITS"
          n490 = local read "MEAS_DCMON"() -> (w1046:bool)
          n491 = local read "ps_meas(i)(w)"() -> (w1054:dbl[])
          n492 = local read "EXT_ATT"() -> (w1028:dbl)
          n493 = case shown="True" w1046 {
            tunnel: [TRUE w1072] -> w1030
            frame False {
            }
            frame True {
              n494 = local read "imon_pass?(t)"() -> (w1072:bool)
            }
          }
          n495 = local read "fsl_ampl_corr"() -> (w1037:dbl)
          n496 = local read "MEAS_PS"() -> (w1045:bool)
          n497 = local read "pout_hsl"() -> (w1038:dbl)
          n498 = local read "dcw_hsl"() -> (w1051:dbl)
          n499 = local read "pout_lsl"() -> (w1039:dbl)
          n500 = local read "dcw_lsl"() -> (w1050:dbl)
          n501 = Equal To 0?(x=w1028) -> (x = 0?=w1027:bool)
          n502 = Index Array(array=w1054, index=1) -> (element=w1052:dbl)
          n503 = case shown="True" w1027 {
            tunnel: w1039 -> [_ w1062]
            tunnel: w1038 -> [_ w1061]
            tunnel: w1037 -> [_ w1060]
            tunnel: [w1056 w1059] -> w1036
            tunnel: [w1056 w1058] -> w1035
            tunnel: [TRUE w1057] -> w1029
            frame False {
              w1056 = "-1"
            }
            frame True {
              n504 = Number To Fractional String(number=w1061) -> (F-format string=w1059:string)  [unwired: 3 in]
              n505 = In Range and Coerce(upper limit=w1061, x=w1060, lower limit=w1062) -> (In Range?=w1057:bool)  [unwired: 1 out]
              n506 = Number To Fractional String(number=w1062) -> (F-format string=w1058:string)  [unwired: 3 in]
            }
          }
          n507 = case shown="True" w1045 {
            tunnel: w1052 -> [_ w1070]
            tunnel: w1051 -> [_ w1069]
            tunnel: w1050 -> [_ w1068]
            tunnel: [w1064 w1067] -> w1049
            tunnel: [w1064 w1066] -> w1048
            tunnel: [TRUE w1065] -> w1031
            frame False {
              w1064 = "-1"
            }
            frame True {
              n508 = Number To Fractional String(number=w1069) -> (F-format string=w1067:string)  [unwired: 3 in]
              n509 = In Range and Coerce(upper limit=w1069, x=w1070, lower limit=w1068) -> (In Range?=w1065:bool)  [unwired: 1 out]
              n510 = Number To Fractional String(number=w1068) -> (F-format string=w1066:string)  [unwired: 3 in]
            }
          }
          n511 = Format Into String(format string="%d", w1029) -> (resulting string=w1034:string)  [unwired: 2 in, 1 out]
          n512 = Format Into String(format string="%d", w1031) -> (resulting string=w1044:string)  [unwired: 2 in, 1 out]
          n513 = Format Into String(format string="%d", w1030) -> (resulting string=w1040:string)  [unwired: 2 in, 1 out]
          n514 = Build Array(w1036, w1035, w1034) -> (w1032:string[])
          n515 = Build Array(w1049, w1048, w1044) -> (w1047:string[])
          n516 = Build Array(w1040) -> (w1041:string[])
        }
      }
      n517 = local read "cmd;"() -> (w942:string)
      n518 = Empty String/Path?(string/path=w942) -> (empty?=w943:bool)
      n519 = Build Array(w948, w947, w946, w944) -> (w949:bool[])
      n520 = And Array Elements(Boolean array=w949) -> (logical AND=w950:bool)
      n521 = case shown="True" w943 {
        tunnel: w942 -> [w961 _]
        tunnel: [w961 "-1" ("cmd;")] -> w941
        frame False {
        }
        frame True {
        }
      }
      n522 = Boolean To (0,1)(Boolean=w950) -> (0, 1=w951:i16)
      n523 = global read "Test Parameter Globals_1.0.0.vi" "Global SN"() -> (w956:string)
      n524 = Format Into String(w951) -> (resulting string=w945:string)  [unwired: 3 in, 1 out]
    }
  }
  n525 = local read "fault?(t)"() -> (w5:bool)
  n526 = local read "temp 0x"() -> (w2:string)
  n527 = Format Into String(format string="%d", w5) -> (resulting string=w3:string)  [unwired: 2 in, 1 out]
  n528 = Insert Into Array(array=w18, new element #1=w14, new element #2=w15, new element #3=w2, new element #4=w10, new element #5=w9, new element #6=w8, new element #7=w7, new element #8=w6, new element #9=w3) -> (→"Payload Results":string[])  [unwired: 1 in]
  "error out" <- w16
